vi "Auto2.vi"() -> ()   [LabVIEW 2020]
uses:
  Global_Variable/A180648.vi
  Global_Variable/Global.vi
  Global_Variable/excursion.vi
  <userlib>/_MGI/1D Array/MGI Running Average/MGI Running Average(DBL).vi
  <userlib>/_MGI/1D Array/MGI Average/MGI Average (DBL[][]).vi
  Libraries/S7/S7.lvlib
  <vilib>/ptbypt/NI_PtbyPt.lvlib
panel:
  out "合格状态":bool
  out "可信度检测":cluster{dbl[], dbl[]}[](graph)
  out "传感器特性":cluster{dbl[], dbl[]}[](graph)
  out "初始角度":dbl
  out "T1-T2_135°":dbl
  out "T1-T2_225°":dbl
  out "T1-T2_315°":dbl
  out "T1-T2_360°":dbl
  out "T1-T2_270°":dbl
  out "T1-T2_180°":dbl
  out "T1-T2_45°":dbl
  out "T1-T2_90°":dbl
  out "初始化 3":bool[](array[boolean])
  out "动优化态前":cluster{dbl[], dbl[]}[](graph)
  in  "initialize 2":bool caption="初始化"
  in  "initialize":bool caption="初始化"
  out "vRES_cCW":cluster{dbl[], dbl[]}
  out "VRES_cW":cluster{dbl[], dbl[]}
  out "初始化 2":bool[](array[boolean])
  in  "选项卡控件":enum32{"工位二程序复检", "工位二动态复检"}(tab)
  in  "请启动":bool
  out "Vres_45°":dbl format="%#.6f"
  out "Vres_135°":dbl format="%#.6f"
  out "Vres_225°":dbl format="%#.6f"
  out "Vres_315°":dbl format="%#.6f"
  out "Vres_360°":dbl format="%#.6f"
  out "Vres_270°":dbl format="%#.6f"
  out "Vres_180°":dbl format="%#.6f"
  out "Vres_90°":dbl format="%#.6f"
  out "S_CCw":dbl[](array[numeric]) caption="数据" format="%0.6f"
  out "P_CCw":dbl[](array[numeric]) caption="数据" format="%0.6f"
  out "S_CW":dbl[](array[numeric]) caption="数据" format="%0.6f"
  out "P_CW":dbl[](array[numeric]) caption="数据" format="%0.6f"
  out "T1_CCw":dbl[](array[numeric]) caption="数据" format="%0.2f"
  out "T2_CCw":dbl[](array[numeric]) caption="数据" format="%0.2f"
  out "T2_CW":dbl[](array[numeric]) caption="数据" format="%0.2f"
  out "T1_CW":dbl[](array[numeric]) caption="数据" format="%0.2f"
  out "初始化":bool[](array[boolean])
  out "SENSOR":T1
  in  "判定结果":bool[][](array[boolean])=[[TRUE]]
  in  "STEP":string
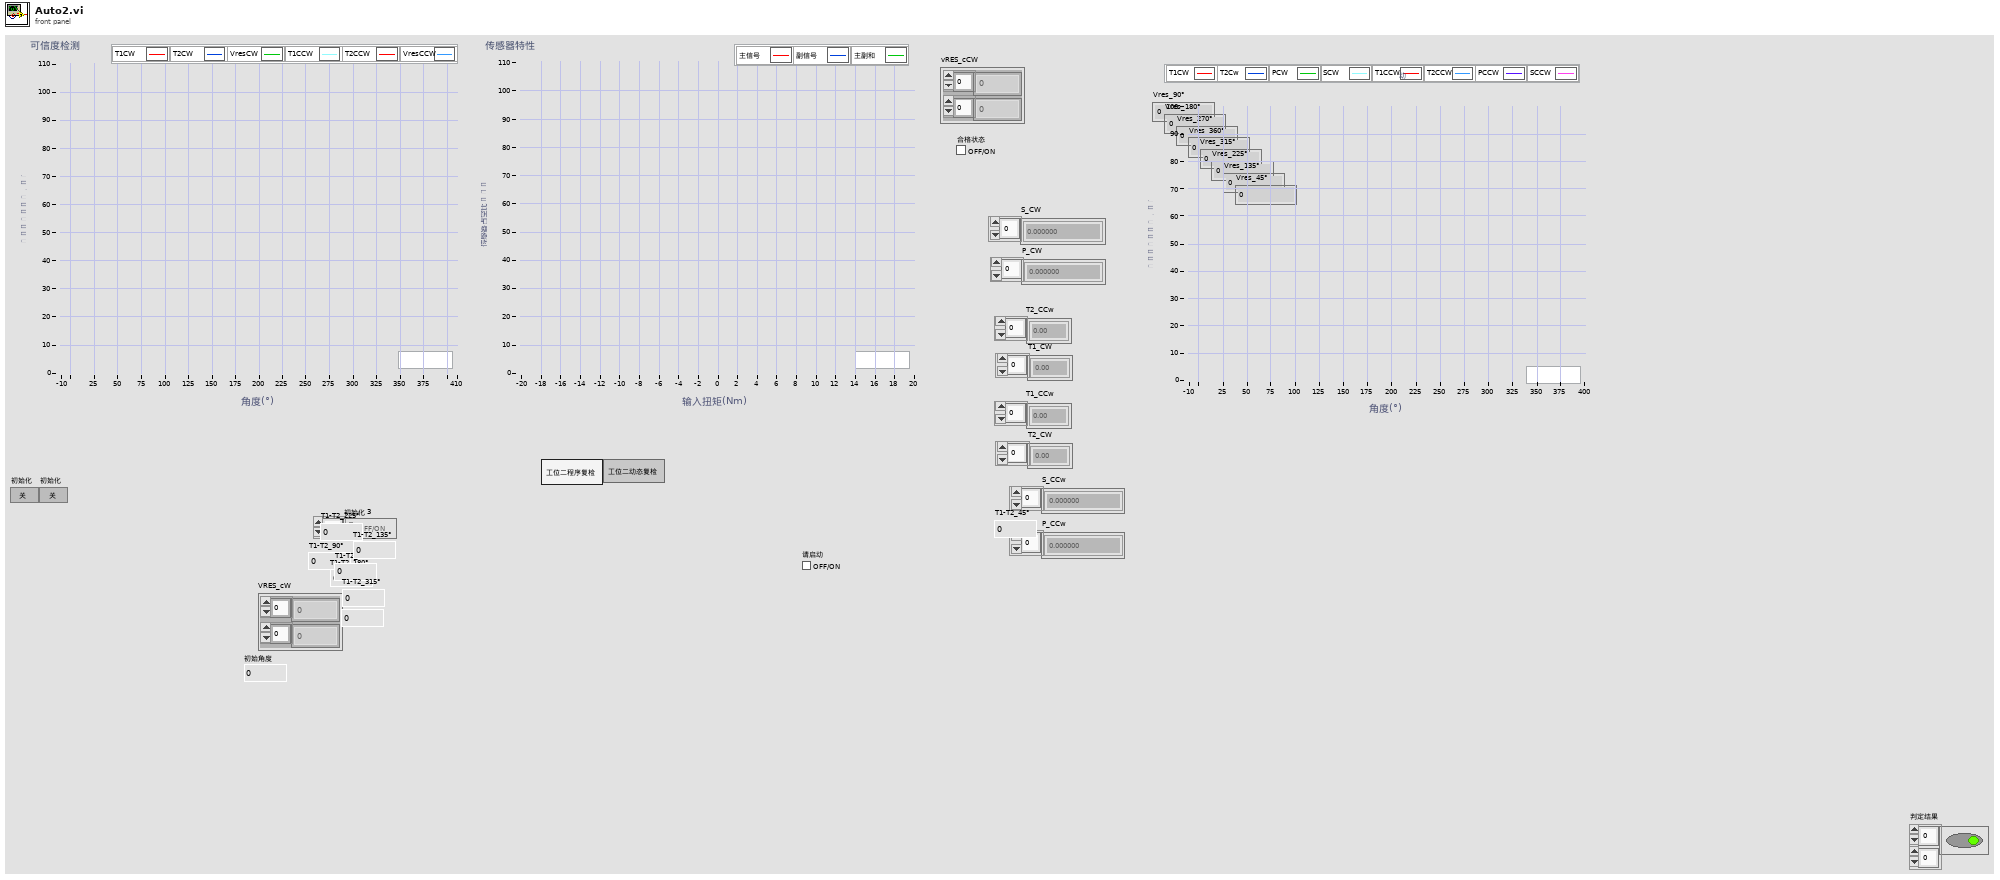
[diagram p1: front panel]
types:
  T1 = cluster{"hSENSOR":i32, "hASIC_T1":i32, "hASIC_T2":i32, "hASIC_P":i32, "hASIC_S":i32}
  T2 = typedef "检测CTR.xctl/检测CTR数据.ctl" = enum16{"Idle", "Runing", "Pass", "Faild", "Skip"}
  T3 = enum32{"Invalid", "Standard", "Closed", "Hidden", "Minimized", "Maximized"}
  T4 = enum16{"Idle", "Runing", "Pass", "Faild", "Skip"}
  T5 = enum16{"open", "replace", "create", "open or create", "replace or create", "replace or create with confirmation"}
  T6 = cluster{"工位一驱动伺服位移":sgl, "工位二驱动伺服位移":sgl, "工位一移载伺服位移":sgl, "工位二移载伺服位移":sgl, "工位一编码器位移":sgl, "工位二编码器位移":sgl, "工位一扭矩":sgl, "工位二扭矩":sgl}
  T7 = typedef "System_conf.ctl" = cluster{"右上升":dbl, "右下降":dbl, "左上升":dbl, "左下降":dbl, "左逆向":dbl, "左正向":dbl}
  T8 = cluster{"主副信号和MAX":cluster{"单位":string, "下限":dbl, "上限":dbl}, "主副信号和MIN":cluster{"单位":string, "下限":dbl, "上限":dbl}, "主信号线性误差":cluster{"单位":string, "下限":dbl, "上限":dbl}, "副信号线性误差":cluster{"单位":string, "下限":dbl, "上限":dbl}, "主信号MAX":cluster{"单位":string, "下限":dbl, "上限":dbl}, "主信号MIN":cluster{"单位":string, "下限":dbl, "上限":dbl}, "副信号MAX":cluster{"单位":string, "下限":dbl, "上限":dbl}, "副信号MIN":cluster{"单位":string, "下限":dbl, "上限":dbl}, "中心偏移量":cluster{"单位":string, "下限":dbl, "上限":dbl}, "定点设置":cluster{"单位":string, "下限":dbl, "上限":dbl}, "定点左侧主信号":cluster{"单位":string, "下限":dbl, "上限":dbl}, "定点左侧副信号":cluster{"单位":string, "下限":dbl, "上限":dbl}, "定点右侧主信号":cluster{"单位":string, "下限":dbl, "上限":dbl}, "定点右侧副信号":cluster{"单位":string, "下限":dbl, "上限":dbl}, "监测点1左滞后":cluster{"单位":string, "下限":dbl, "上限":dbl}, "监测点1右滞后":cluster{"单位":string, "下限":dbl, "上限":dbl}, "监测点2左滞后":cluster{"单位":string, "下限":dbl, "上限":dbl}, "监测点2右滞后":cluster{"单位":string, "下限":dbl, "上限":dbl}, "监测点3左滞后":cluster{"单位":string, "下限":dbl, "上限":dbl}, "监测点3右滞后":cluster{"单位":string, "下限":dbl, "上限":dbl}}
  T9 = cluster{"复检速度":dbl, "换向扭矩":dbl, "判定范围下限":dbl, "判定范围上限":dbl, "滞后监测点1":dbl, "滞后监测点2":dbl, "滞后监测点3":dbl}
  T10 = cluster{"可信度检测":cluster{dbl[], dbl[]}[], "动优化态前":cluster{dbl[], dbl[]}[], "传感器特性":cluster{dbl[], dbl[]}[]}
  T11 = typedef "lveventtype.ctl" = enum32{"Null", "Timeout", "Annotation Menu Selection", "Annotation Menu Selection?", "App Instance Close", "App Instance Close?", "Autoscale Range Change", "Bookmark Info Change", "Cell Edit", "Cell Edit?", "Cursor Grab", "Cursor Grab?", "Cursor Menu Selection", "Cursor Menu Selection?", "Cursor Move", "Cursor Release", "Data Change", "Direction Change", "Display State Change", "Drag Ended", "Drag Enter", "Drag Leave", "Drag Over", "Drag Source Update", "Drag Starting", "Drag Starting?", "Drop", "Exec State Change", "Key Down", "Key Down?", "Key Repeat", "Key Repeat?", "Key Up", "Listbox Double Click", "Menu Activation?", "Menu Selection (App)", "Menu Selection? (App)", "Menu Selection (User)", "Mouse Down", "Mouse Down?", "Mouse Enter", "Mouse Leave", "Mouse Move", "Mouse Up", "Mouse Wheel", "NI Security User Change (App)", "Pane Size", "Panel Close", "Panel Close?", "Panel Resize", "Plot Attribute Change", "Scale Range Change", "Shortcut Menu Activation?", "Shortcut Menu Selection (App)", "Shortcut Menu Selection? (App)", "Shortcut Menu Selection (User)", "Tree Double Click", "Tree Drag", "Tree Drag?", "Tree Drop", "Tree Drop?", "Tree Item Close", "Tree Item Close?", "Tree Item Open", "Tree Item Open?", "User Event", "Value Change"}
  T12 = typedef "LVPoint32TypeDef.ctl" = cluster{"Horizontal":i32, "Vertical":i32}
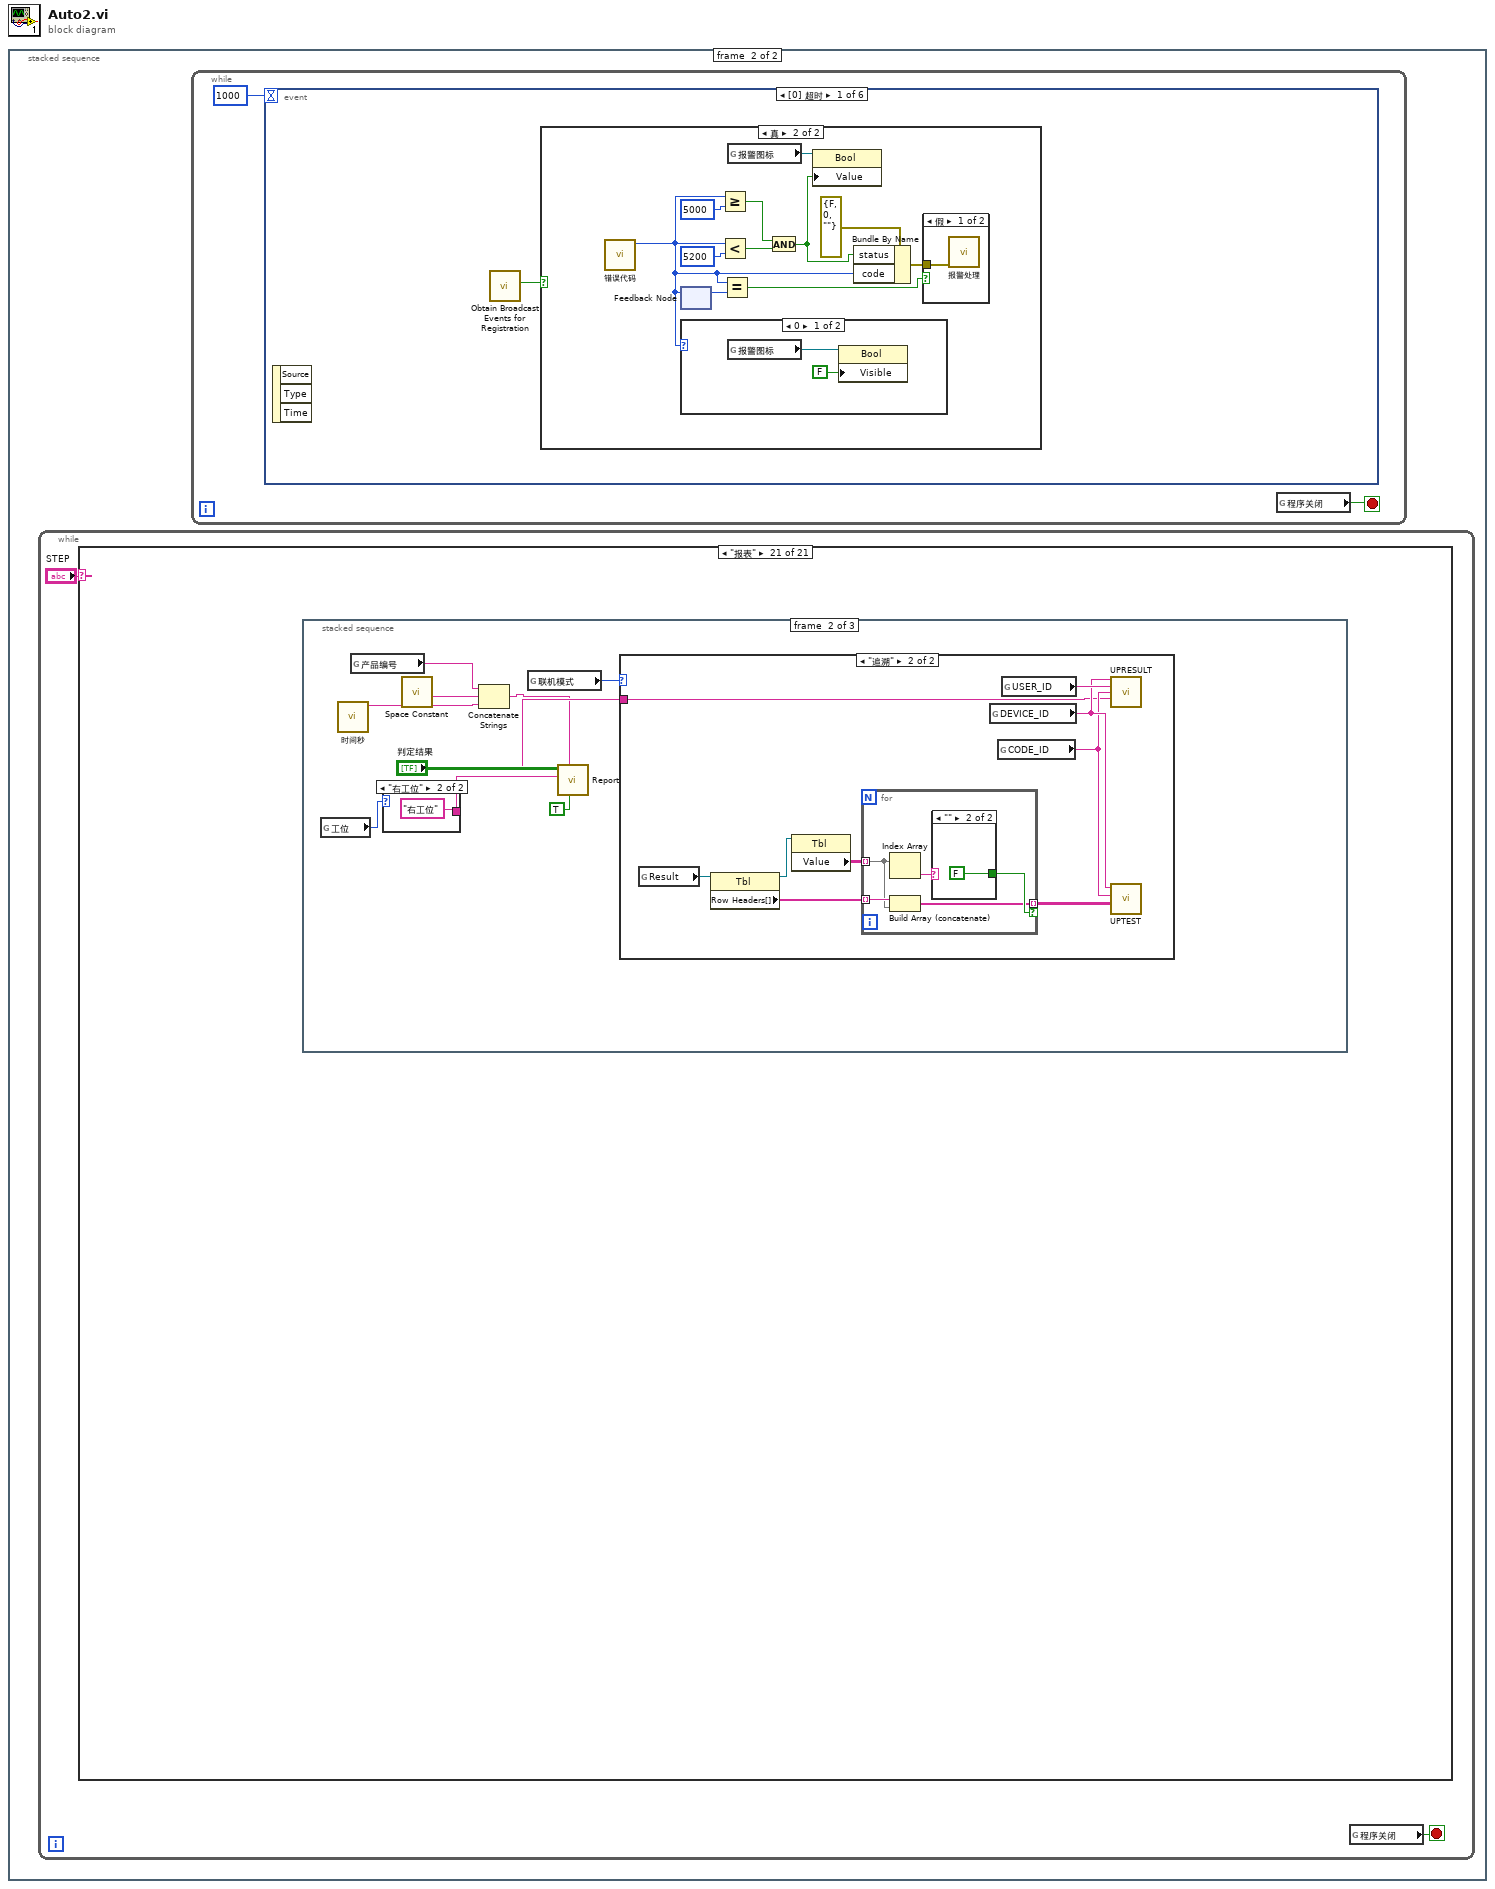
[diagram p0: block diagram]
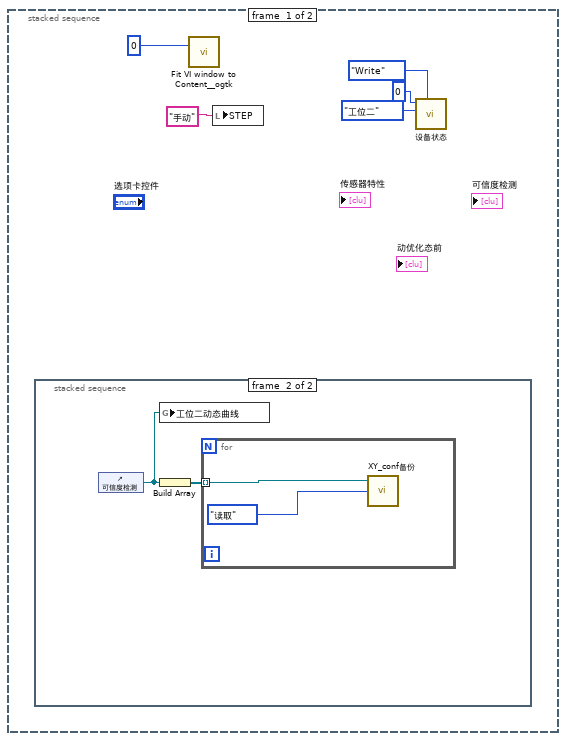
[diagram p2: hidden frame]
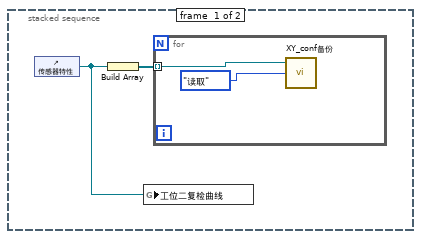
[diagram p3: hidden frame]
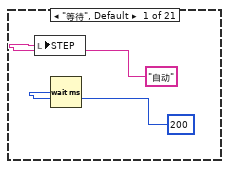
[diagram p4: hidden frame]
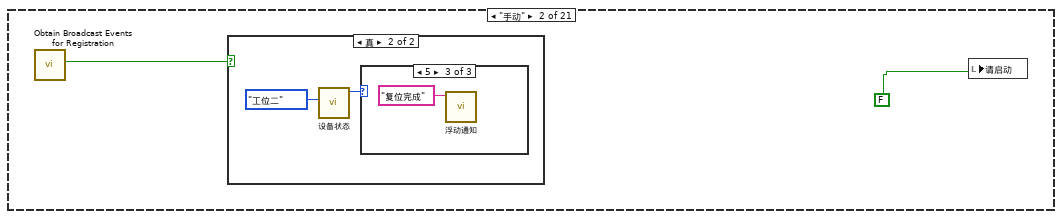
[diagram p5: hidden frame]
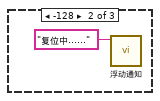
[diagram p8: hidden frame]
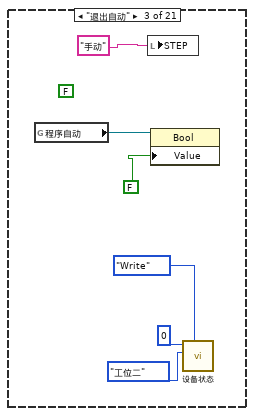
[diagram p9: hidden frame]
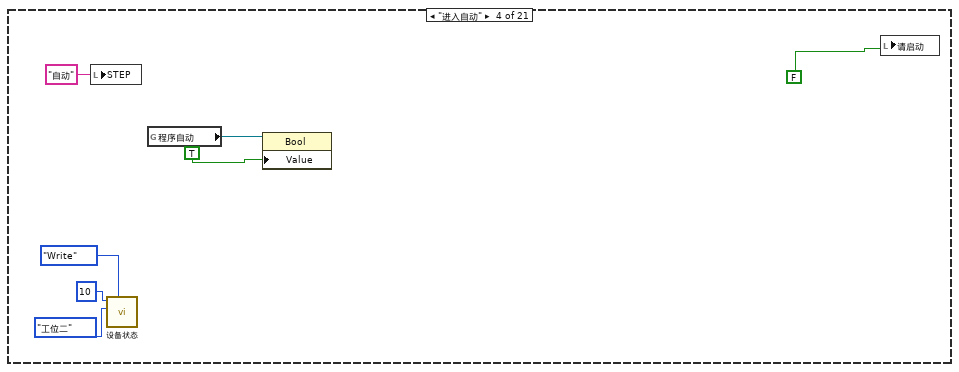
[diagram p10: hidden frame]
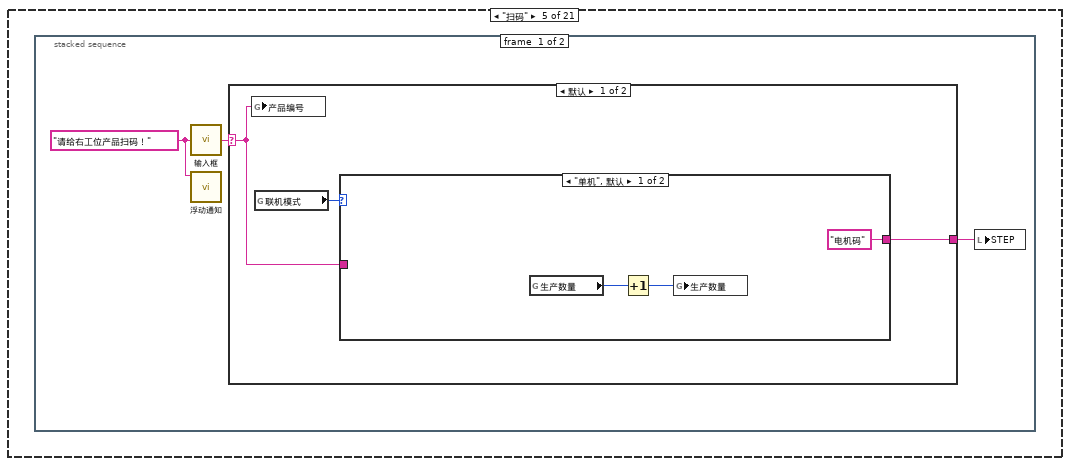
[diagram p11: hidden frame]
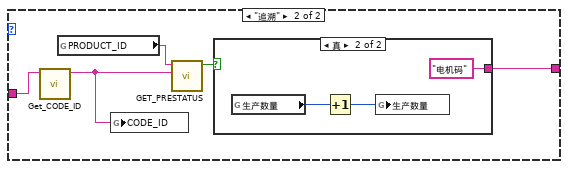
[diagram p12: hidden frame]
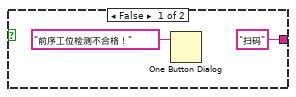
[diagram p13: hidden frame]
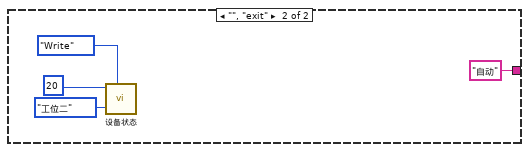
[diagram p14: hidden frame]
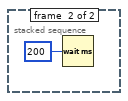
[diagram p15: hidden frame]
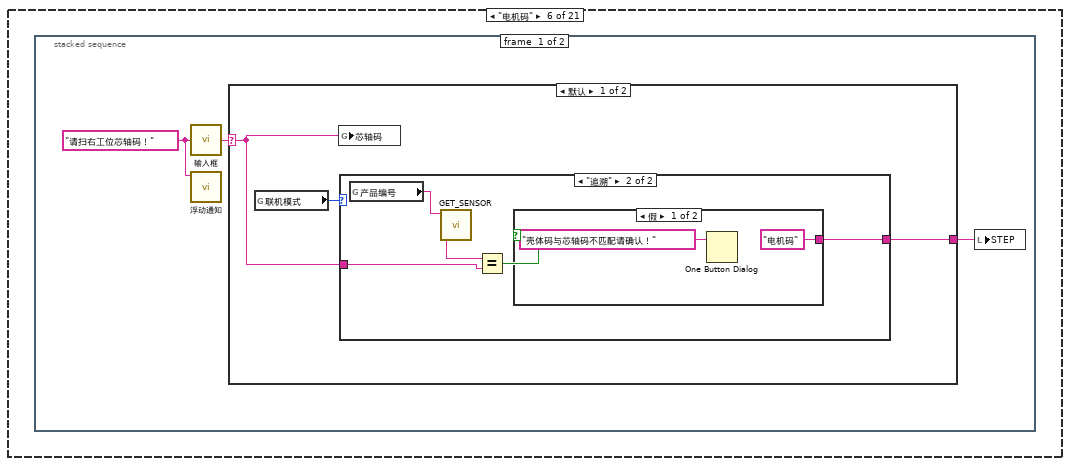
[diagram p16: hidden frame]
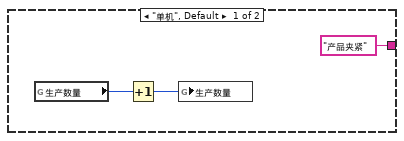
[diagram p17: hidden frame]
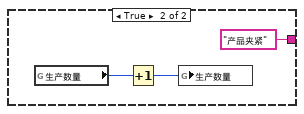
[diagram p18: hidden frame]
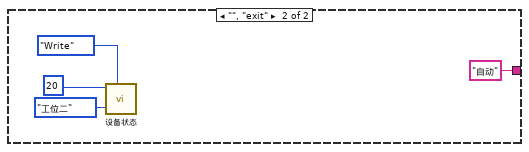
[diagram p19: hidden frame]
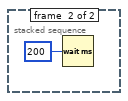
[diagram p20: hidden frame]
diagram:
  n1 = stacked-sequence {
    frame #0 {
      n2 = stacked-sequence {
        frame #0 {
          n3 = control-ref of="传感器特性"() -> (w6:refnum<vi>)
          n4 = Build Array(w6) -> (w7:refnum<vi>[])
          n5 = global write "A180648.vi" "工位二复检曲线"(w6) -> ()
          n6 = for "For循环" {
            tunnel: w7 -> [w8] mode=indexing
            n7 = call "XY_conf备份.vi"("方式"=enum16{"写入", "读取"}."读取", "XY图引用"=w8) -> ()  [unwired: 3 in, 1 out]
          }
        }
        frame #1 {
          n8 = control-ref of="可信度检测"() -> (w11:refnum<vi>)
          n9 = global write "A180648.vi" "工位二动态曲线"(w11) -> ()
          n10 = Build Array(w11) -> (w10:refnum<vi>[])
          n11 = for "For循环" {
            tunnel: w10 -> [w12] mode=indexing
            n12 = call "XY_conf备份.vi"("方式"=enum16{"写入", "读取"}."读取", "XY图引用"=w12) -> ()  [unwired: 3 in, 1 out]
          }
        }
      }
      n13 = call <userlib>:"Fit VI window to Content__ogtk.vi"("border spacing (2 px)"=0) -> ()  [unwired: 5 in, 2 out]
      n14 = local write "STEP"("手动" ("STEP")) -> ()
      n15 = call "设备状态.vi"("枚举"=enum16{"Read", "Write"}."Write", "工位"=enum16{"工位一", "工位二"}."工位二", "Status_Write"=i16 0) -> ()  [unwired: 8 in, 1 out]
    }
    frame #1 {
      n16 = while {
        stop <- w15 stop-if-true
        n17 = case shown="\"报表\"" "STEP" {
          frame "等待", Default {
            n18 = local write "STEP"("自动" ("STEP")) -> ()
            n19 = Wait (ms)(milliseconds to wait=u32 200 ("等待时间（毫秒）")) -> ()  [unwired: 1 out]
          }
          frame "手动" {
            n20 = call "Obtain Broadcast Events for Registration.vi"() -> ("Already running?"=w19:bool)  [unwired: 9 in, 2 out]
            n21 = case shown="真" w19 {
              frame False {
              }
              frame True {
                n22 = call "设备状态.vi"("工位"=enum16{"工位一", "工位二"}."工位二") -> ("Status_Read"=w21:i16)  [unwired: 10 in]
                n23 = case shown="5" w21 {
                  frame 0, Default {
                  }
                  frame -128 {
                    n24 = call "浮动通知.vi"("通知内容"="复位中……" ("Status")) -> ()  [unwired: 11 in]
                  }
                  frame 5 {
                    n25 = call "浮动通知.vi"("通知内容"="复位完成" ("Status")) -> ()  [unwired: 11 in]
                  }
                }
              }
            }
            n26 = local write "请启动"(FALSE ("请启动")) -> ()
          }
          frame "退出自动" {
            (unwired) FALSE ("计时开始")
            n27 = global read "Global.vi" "程序自动"() -> (w26:refnum<vi>)
            n28 = local write "STEP"("手动" ("STEP")) -> ()
            n29 = property class="Bool"(reference=w26, "Value"=FALSE) -> ()  [unwired: 1 in, 2 out]
            n30 = call "设备状态.vi"("枚举"=enum16{"Read", "Write"}."Write", "工位"=enum16{"工位一", "工位二"}."工位二", "Status_Write"=i16 0) -> ()  [unwired: 8 in, 1 out]
          }
          frame "进入自动" {
            n31 = local write "STEP"("自动" ("STEP")) -> ()
            n32 = call "设备状态.vi"("枚举"=enum16{"Read", "Write"}."Write", "工位"=enum16{"工位一", "工位二"}."工位二", "Status_Write"=i16 10) -> ()  [unwired: 8 in, 1 out]
            n33 = global read "Global.vi" "程序自动"() -> (w35:refnum<vi>)
            n34 = property class="Bool"(reference=w35, "Value"=TRUE) -> ()  [unwired: 1 in, 2 out]
            n35 = local write "请启动"(FALSE ("请启动")) -> ()
          }
          frame "扫码" {
            n36 = stacked-sequence {
              frame #0 {
                w38 = "请给右工位产品扫码！" ("提示信息")
                n37 = call "输入框.vi"("提示信息"=w38) -> ("条形码输出"=w39:string)
                n38 = call "浮动通知.vi"("通知内容"=w38) -> ()  [unwired: 11 in]
                n39 = case shown="默认" w39 {
                  selector: w39 -> [w40 _]
                  tunnel: [w42 "自动" ("State(s) in Front (\"\")")] -> w37
                  frame Default {
                    n40 = global write "Global.vi" "产品编号"(w40) -> ()
                    n41 = global read "Global.vi" "联机模式"() -> (w41:enum16{"单机", "追溯"})
                    n42 = case shown="\"单机\", 默认" w41 {
                      tunnel: ["电机码" ("State(s) in Front (\"\")") w50] -> w42
                      tunnel: w40 -> [_ w47]
                      frame "单机", Default {
                        n43 = global read "Global.vi" "生产数量"() -> (w43:i32)
                        n44 = Increment(x=w43) -> (x+1=w44:i32)
                        n45 = global write "Global.vi" "生产数量"(w44) -> ()
                      }
                      frame "追溯" {
                        n46 = call "Get_CODE_ID.vi"("CODE_MAIN"=w47) -> ("CODE_ID"=w46:string)  [unwired: 10 in]
                        n47 = global read "追溯Global.vi" "PRODUCT_ID"() -> (w49:string)
                        n48 = global write "追溯Global.vi" "CODE_ID"(w46) -> ()
                        n49 = call "GET_PRESTATUS.vi"("CODE_ID"=w46, "PRODUCT_ID"=w49) -> ("OK?"=w48:bool)  [unwired: 9 in]
                        n50 = case shown="真" w48 {
                          tunnel: ["扫码" ("State(s) in Front (\"\")") "电机码" ("State(s) in Front (\"\")")] -> w50
                          frame False {
                            n51 = One Button Dialog(message="前序工位检测不合格！" ("消息")) -> ()  [unwired: 1 in, 1 out]
                          }
                          frame True {
                            n52 = global read "Global.vi" "生产数量"() -> (w53:i32)
                            n53 = Increment(x=w53) -> (x+1=w54:i32)
                            n54 = global write "Global.vi" "生产数量"(w54) -> ()
                          }
                        }
                      }
                    }
                  }
                  frame "", "exit" {
                    n55 = call "设备状态.vi"("枚举"=enum16{"Read", "Write"}."Write", "工位"=enum16{"工位一", "工位二"}."工位二", "Status_Write"=i16 20) -> ()  [unwired: 8 in, 1 out]
                  }
                }
                n56 = local write "STEP"(w37) -> ()
              }
              frame #1 {
                n57 = Wait (ms)(milliseconds to wait=u32 200 ("等待时间（毫秒）")) -> ()  [unwired: 1 out]
              }
            }
          }
          frame "电机码" {
            n58 = stacked-sequence {
              frame #0 {
                w62 = "请扫右工位芯轴码！" ("提示信息")
                n59 = call "输入框.vi"("提示信息"=w62) -> ("条形码输出"=w63:string)
                n60 = call "浮动通知.vi"("通知内容"=w62) -> ()  [unwired: 11 in]
                n61 = case shown="默认" w63 {
                  selector: w63 -> [w64 _]
                  tunnel: [w66 "自动" ("State(s) in Front (\"\")")] -> w61
                  frame Default {
                    n62 = global read "Global.vi" "联机模式"() -> (w65:enum16{"单机", "追溯"})
                    n63 = global write "Global.vi" "芯轴码"(w64) -> ()
                    n64 = case shown="\"追溯\"" w65 {
                      tunnel: ["产品夹紧" ("State(s) in Front (\"\")") w74] -> w66
                      tunnel: w64 -> [_ w72]
                      frame "单机", Default {
                        n65 = global read "Global.vi" "生产数量"() -> (w67:i32)
                        n66 = Increment(x=w67) -> (x+1=w68:i32)
                        n67 = global write "Global.vi" "生产数量"(w68) -> ()
                      }
                      frame "追溯" {
                        n68 = global read "Global.vi" "产品编号"() -> (w70:string)
                        n69 = call "GET_SENSOR.vi"("CODE_MAIN"=w70) -> ("CODE_MOTOR"=w73:string)  [unwired: 10 in]
                        n70 = Equal?(x=w73, y=w72) -> (x = y?=w71:bool)
                        n71 = case shown="假" w71 {
                          tunnel: ["电机码" ("State(s) in Front (\"\")") "产品夹紧" ("State(s) in Front (\"\")")] -> w74
                          frame False {
                            n72 = One Button Dialog(message="壳体码与芯轴码不匹配请确认！" ("消息")) -> ()  [unwired: 1 in, 1 out]
                          }
                          frame True {
                            n73 = global read "Global.vi" "生产数量"() -> (w77:i32)
                            n74 = Increment(x=w77) -> (x+1=w78:i32)
                            n75 = global write "Global.vi" "生产数量"(w78) -> ()
                          }
                        }
                      }
                    }
                  }
                  frame "", "exit" {
                    n76 = call "设备状态.vi"("枚举"=enum16{"Read", "Write"}."Write", "工位"=enum16{"工位一", "工位二"}."工位二", "Status_Write"=i16 20) -> ()  [unwired: 8 in, 1 out]
                  }
                }
                n77 = local write "STEP"(w61) -> ()
              }
              frame #1 {
                n78 = Wait (ms)(milliseconds to wait=u32 200 ("等待时间（毫秒）")) -> ()  [unwired: 1 out]
              }
            }
          }
          frame "传感器码" {
            n79 = stacked-sequence {
              frame #0 {
                w86 = "请给右工位产品扫码！" ("提示信息")
                n80 = call "输入框.vi"("提示信息"=w86) -> ("条形码输出"=w87:string)
                n81 = call "浮动通知.vi"("通知内容"=w86) -> ()  [unwired: 11 in]
                n82 = case shown="默认" w87 {
                  selector: w87 -> [w88 _]
                  tunnel: [w90 "自动" ("State(s) in Front (\"\")")] -> w85
                  frame Default {
                    n83 = global write "Global.vi" "产品编号"(w88) -> ()
                    n84 = global read "Global.vi" "联机模式"() -> (w89:enum16{"单机", "追溯"})
                    n85 = case shown="\"追溯\"" w89 {
                      tunnel: ["产品夹紧" ("State(s) in Front (\"\")") w98] -> w90
                      tunnel: w88 -> [_ w95]
                      frame "单机", Default {
                        n86 = global read "Global.vi" "生产数量"() -> (w91:i32)
                        n87 = Increment(x=w91) -> (x+1=w92:i32)
                        n88 = global write "Global.vi" "生产数量"(w92) -> ()
                      }
                      frame "追溯" {
                        n89 = call "Get_CODE_ID_Sensor.vi"("CODE_SENSOR"=w95) -> ("CODE_ID"=w94:string)  [unwired: 10 in]
                        n90 = global read "追溯Global.vi" "PRODUCT_ID"() -> (w97:string)
                        n91 = global write "追溯Global.vi" "CODE_ID"(w94) -> ()
                        n92 = call "GET_PRESTATUS.vi"("CODE_ID"=w94, "PRODUCT_ID"=w97) -> ("OK?"=w96:bool)  [unwired: 9 in]
                        n93 = case shown="假" w96 {
                          tunnel: ["传感器码" ("State(s) in Front (\"\")") "产品夹紧" ("State(s) in Front (\"\")")] -> w98
                          frame False {
                            n94 = One Button Dialog(message="前序工位检测不合格！" ("消息")) -> ()  [unwired: 1 in, 1 out]
                          }
                          frame True {
                            n95 = global read "Global.vi" "生产数量"() -> (w101:i32)
                            n96 = Increment(x=w101) -> (x+1=w102:i32)
                            n97 = global write "Global.vi" "生产数量"(w102) -> ()
                          }
                        }
                      }
                    }
                  }
                  frame "", "exit" {
                    n98 = call "设备状态.vi"("枚举"=enum16{"Read", "Write"}."Write", "工位"=enum16{"工位一", "工位二"}."工位二", "Status_Write"=i16 20) -> ()  [unwired: 8 in, 1 out]
                  }
                }
                n99 = local write "STEP"(w85) -> ()
              }
              frame #1 {
                n100 = Wait (ms)(milliseconds to wait=u32 200 ("等待时间（毫秒）")) -> ()  [unwired: 1 out]
              }
            }
          }
          frame "产品夹紧" {
            n101 = stacked-sequence {
              frame #0 {
                n102 = case shown="假" "请启动" {
                  frame False {
                    n103 = call "浮动通知.vi"("通知内容"="请启动右工位" ("Status")) -> ()  [unwired: 11 in]
                    n104 = call "设备状态.vi"("枚举"=enum16{"Read", "Write"}."Write", "工位"=enum16{"工位一", "工位二"}."工位二", "Status_Write"=i16 99) -> ()  [unwired: 8 in, 1 out]
                    n105 = local write "请启动"(TRUE ("请启动")) -> ()
                  }
                  frame True {
                  }
                }
              }
              frame #1 {
                n106 = call "设备状态.vi"("工位"=enum16{"工位一", "工位二"}."工位二") -> ("Status_Read"=w115:i16)  [unwired: 10 in]
                n107 = case shown="0, 默认" w115 {
                  frame 0, Default {
                  }
                  frame 100 {
                    n108 = local write "STEP"("初始化") -> ()
                    n109 = local write "请启动"(FALSE ("请启动")) -> ()
                  }
                }
              }
            }
          }
          frame "套输入轴" {
            n110 = global read "Global.vi" "可信度检测引用句柄"() -> (w125:refnum<vi>)
            n111 = global read "Global.vi" "传感器特性用句柄"() -> (w128:refnum<vi>)
            n112 = property class="检测CTR"(reference=w125) -> ("Value"=w126:variant)  [unwired: 1 in, 2 out]
            n113 = property class="检测CTR"(reference=w128) -> ("Value"=w127:variant)  [unwired: 1 in, 2 out]
            n114 = Variant To Data(type=检测CTR数据."Idle" ("Data"), Variant=w126) -> (data=w124:T2)  [unwired: 1 in, 1 out]
            n115 = Variant To Data(type=检测CTR数据."Idle" ("Data"), Variant=w127) -> (data=w129:T2)  [unwired: 1 in, 1 out]
            n116 = Equal?(x=w124, y=检测CTR数据."Skip" ("Data")) -> (x = y?=w130:bool)
            n117 = Equal?(x=w129, y=检测CTR数据."Skip" ("Data")) -> (x = y?=w131:bool)
            n118 = And(x=w130, y=w131) -> (x .and. y?=w119:bool)
            n119 = case shown="假" w119 {
              frame False {
                n120 = stacked-sequence {
                  frame #0 {
                    n121 = call "浮动通知.vi"("通知内容"="右工位产品套输入轴" ("Status")) -> ()  [unwired: 11 in]
                    n122 = call "设备状态.vi"("枚举"=enum16{"Read", "Write"}."Write", "工位"=enum16{"工位一", "工位二"}."工位二", "Status_Write"=i16 112) -> ()  [unwired: 8 in, 1 out]
                    n123 = vi-ref "T1T2占空比.vi"() -> (w135:refnum<vi>)
                    n124 = call "CallVI.vi"("VI引用"=w135, "状态"=T3."Hidden") -> ()  [unwired: 12 in, 2 out]
                    n125 = vi-ref "PS采集.vi"() -> (w132:refnum<vi>)
                    n126 = call "CallVI.vi"("VI引用"=w132, "状态"=T3."Hidden") -> ()  [unwired: 12 in, 2 out]
                  }
                  frame #1 {
                    n127 = while {
                      stop <- w140 stop-if-true
                      n128 = call "设备状态.vi"("工位"=enum16{"工位一", "工位二"}."工位二") -> ("Status_Read"=w141:i16)  [unwired: 10 in]
                      n129 = case shown="0, 默认" w141 {
                        tunnel: [w143 TRUE] -> w140
                        frame 0, Default {
                          n130 = call "套输入轴时间"() -> ("Time has Elapsed"=w144:bool)  [unwired: 12 in, 7 out]
                          n131 = case shown="真" w144 {
                            tunnel: [FALSE TRUE] -> w143
                            frame False {
                            }
                            frame True {
                              n132 = call "浮动通知.vi"("通知内容"="工位二产品套输入轴超时" ("Status")) -> ()  [unwired: 11 in]
                            }
                          }
                        }
                        frame 113 {
                          n133 = local write "STEP"("动态优化") -> ()
                        }
                      }
                    }
                  }
                }
              }
              frame True {
                n134 = local write "STEP"("程序固化" ("STEP")) -> ()
              }
            }
          }
          frame "套输出轴" {
            n135 = global read "Global.vi" "传感器特性用句柄"() -> (w155:refnum<vi>)
            n136 = property class="检测CTR"(reference=w155) -> ("Value"=w154:variant)  [unwired: 1 in, 2 out]
            n137 = Variant To Data(type=检测CTR数据."Idle" ("Data"), Variant=w154) -> (data=w156:T2)  [unwired: 1 in, 1 out]
            n138 = Equal?(x=w156, y=检测CTR数据."Skip" ("Data")) -> (x = y?=w151:bool)
            n139 = case shown="假" w151 {
              frame False {
                n140 = stacked-sequence {
                  frame #0 {
                    n141 = call "设备状态.vi"("枚举"=enum16{"Read", "Write"}."Write", "工位"=enum16{"工位一", "工位二"}."工位二", "Status_Write"=i16 108) -> ()  [unwired: 8 in, 1 out]
                    n142 = call "浮动通知.vi"("通知内容"="右工位产品套输出轴" ("Status")) -> ()  [unwired: 11 in]
                  }
                  frame #1 {
                    n143 = while {
                      stop <- w161 stop-if-true
                      n144 = call "设备状态.vi"("工位"=enum16{"工位一", "工位二"}."工位二") -> ("Status_Read"=w162:i16)  [unwired: 10 in]
                      n145 = case shown="0, 默认" w162 {
                        tunnel: [w164 TRUE] -> w161
                        frame 0, Default {
                          n146 = call "套输出轴时间"() -> ("Time has Elapsed"=w165:bool)  [unwired: 12 in, 7 out]
                          n147 = case shown="真" w165 {
                            tunnel: [FALSE TRUE] -> w164
                            frame False {
                            }
                            frame True {
                              n148 = call "浮动通知.vi"("通知内容"="右工位产品套输出轴超时" ("Status")) -> ()  [unwired: 11 in]
                            }
                          }
                        }
                        frame 109 {
                          n149 = call "传感器数据.vi"() -> ("传感器读数"=w170:T6)  [unwired: 11 in]
                          n150 = local write "STEP"("程序复检") -> ()
                          n151 = Unbundle By Name(w170) -> ("工位二驱动伺服位移"=→"初始角度":sgl)
                        }
                      }
                    }
                  }
                }
              }
              frame True {
                n152 = local read "判定结果"() -> (w174:bool[][])
                n153 = Build Array (concatenate)(w174, bool[][] [[FALSE, TRUE]] ("判定结果")) -> (w175:bool[][])
                n154 = local write "判定结果"(w175) -> ()
                n155 = local write "STEP"("程序固化" ("STEP")) -> ()
              }
            }
          }
          frame "初始化" {
            n156 = stacked-sequence {
              frame #0 {
                w182 = cluster{dbl[], dbl[]} {[], []} ("vRES_cCW")
                w180 = TRUE ("IO_Stop")
                n157 = global read "Global.vi" "产品型号"() -> (w178:string)
                n158 = global write "Global.vi" "IO_Stop"(w180) -> ()
                n159 = global write "Global.vi" "计时开始"(w180) -> ()
                n160 = global write "Global.vi" "工位占空比采集"(FALSE ("工位二占空比采集")) -> ()
                n161 = global write "Global.vi" "P/S采集"(FALSE ("工位二占空比采集")) -> ()
                n162 = local write "判定结果"(bool[][] [] ("判定结果")) -> ()
                n163 = call "System_Conf_RW.vi"("Mode"=enum16{"Read", "Write"}."Read", "Section"=w178) -> ("excursion_out"=w177:T7)  [unwired: 8 in, 1 out]
                n164 = global write "excursion.vi" "excursion"(w177) -> ()
                n165 = global write "Global.vi" "动态优化完成"(FALSE ("动态优化完成")) -> ()
                n166 = local write "vRES_cCW"(w182) -> ()
                n167 = local write "VRES_cW"(w182) -> ()
              }
              frame #1 {
                w191 = dbl[] [] ("S_CCw")
                w192 = dbl[] [] ("T1_cw")
                n168 = local write "T1_CW"(w192) -> ()
                n169 = local write "T2_CW"(w192) -> ()
                n170 = local write "P_CW"(w192) -> ()
                n171 = local write "P_CCw"(w192) -> ()
                n172 = for "For循环" {
                  N: 12 -> [_]
                  tunnel: [cluster{dbl[], dbl[]} {[], []}] -> w190 mode=indexing
                }
                n173 = local write "传感器特性"(w190) -> ()
                n174 = local write "S_CCw"(w191) -> ()
                n175 = local write "S_CW"(w191) -> ()
                n176 = local write "T1_CCw"(w191) -> ()
                n177 = local write "T2_CCw"(w191) -> ()
                n178 = for "For循环" {
                  N: 8 -> [_]
                  tunnel: [cluster{dbl[], dbl[]} {[], []}] -> w188 mode=indexing
                }
                n179 = for "For循环" {
                  N: 8 -> [_]
                  tunnel: [cluster{dbl[], dbl[]} {[], []}] -> w187 mode=indexing
                }
                n180 = local write "动优化态前"(w187) -> ()
                n181 = local write "可信度检测"(w188) -> ()
              }
              frame #2 {
                n182 = global read "Global.vi" "Result"() -> (w208:refnum<vi>)
                n183 = property class="Tbl"(reference=w208, "Value"=string[][] []) -> (reference out=w209:refnum<vi>, error out=w210:errorcluster)  [unwired: 1 in]
                n184 = property class="Tbl"(reference=w209, error in=w210, "Row Headers[]"=string[] [] ("列首字符串[]")) -> ()  [unwired: 2 out]
                n185 = Initialize Array(TRUE, 12 ("维数大小")) -> (→"初始化":bool[])
                n186 = Initialize Array(TRUE, 8 ("维数大小")) -> (→"初始化 2":bool[])
                n187 = Initialize Array(TRUE, 8 ("维数大小")) -> (→"初始化 3":bool[])
              }
              frame #3 {
                n188 = global read "Global.vi" "传感器特性用句柄"() -> (w214:refnum<vi>)
                n189 = global read "Global.vi" "可信度检测引用句柄"() -> (w211:refnum<vi>)
                n190 = global read "Global.vi" "动态优化引用句柄"() -> (w212:refnum<vi>)
                n191 = global read "Global.vi" "静态标定引用句柄"() -> (w216:refnum<vi>)
                n192 = global read "Global.vi" "程序固化引用句柄"() -> (w215:refnum<vi>)
                n193 = Build Array(w216, w215, w214, w212, w211) -> (w213:refnum<vi>[])
                n194 = for "For循环" {
                  tunnel: w213 -> [w226] mode=indexing
                  n195 = property class="检测CTR"(reference=w226) -> (reference out=w225:refnum<vi>, "Value"=w224:variant)  [unwired: 1 in, 1 out]
                  n196 = Variant To Data(type=检测CTR数据."Idle" ("Data"), Variant=w224) -> (data=w222:T2)  [unwired: 1 in, 1 out]
                  n197 = Equal?(x=w222, y=检测CTR数据."Skip" ("Data")) -> (x = y?=w220:bool)
                  n198 = Select(t=检测CTR数据."Skip" ("Data"), s=w220, f=检测CTR数据."Idle" ("Data")) -> (s? t:f=w217:T2)
                  n199 = property class="检测CTR"(reference=w225, "Value"=w217) -> ()  [unwired: 1 in, 2 out]
                }
              }
              frame #4 {
                n200 = local write "STEP"("静态标定" ("STEP")) -> ()
              }
            }
          }
          frame "静态标定" {
            n201 = global read "Global.vi" "静态标定引用句柄"() -> (w232:refnum<vi>)
            n202 = property class="检测CTR"(reference=w232) -> ("Value"=w231:variant)  [unwired: 1 in, 2 out]
            n203 = Variant To Data(type=检测CTR数据."Idle" ("Data"), Variant=w231) -> (data=w233:T2)  [unwired: 1 in, 1 out]
            n204 = Equal?(x=w233, y=检测CTR数据."Skip" ("Data")) -> (x = y?=w228:bool)
            n205 = case shown="真" w228 {
              frame False {
                n206 = stacked-sequence {
                  tunnel: [_ _ w250] -> w234
                  frame #0 {
                    n207 = global read "Global.vi" "静态标定引用句柄"() -> (w236:refnum<vi>)
                    n208 = call "浮动通知.vi"("通知内容"="静态标定" ("Status")) -> ()  [unwired: 11 in]
                    n209 = property class="检测CTR"(reference=w236, "Value"=T4."Runing" ("值")) -> ()  [unwired: 1 in, 2 out]
                  }
                  frame #1 {
                    n210 = flat-sequence {
                      frame #0 {
                        n211 = call "采集切换.vi"("工位"=enum16{"工位一", "工位二"}."工位二", "采集方式"=enum16{"板卡采集", "PGI采集"}."PGI采集") -> ()  [unwired: 10 in]
                      }
                      frame #1 {
                        n212 = Wait (ms)(milliseconds to wait=u32 100 ("等待时间（毫秒）")) -> ()  [unwired: 1 out]
                      }
                    }
                  }
                  frame #2 {
                    n213 = call "InitPGI.vi"("DeviceNumber"=1) -> ("SENSOR"=w242:T1, "error out"=w243:errorcluster)  [unwired: 13 in]
                    "SENSOR" <- w242
                    n214 = call "InitProduct.vi"("SENSOR"=w242, "error in (no error)"=w243) -> ("error out"=w241:errorcluster)  [unwired: 12 in, 1 out]
                    n215 = call "StaticCalibration改.vi"("SENSOR"=w242, "error in (no error)"=w241) -> ("OK？"=w245:bool, "error out"=w247:errorcluster)  [unwired: 9 in, 3 out]
                    n216 = call "浮动通知.vi"("通知内容"="静态标定中..." ("Status")) -> ()  [unwired: 11 in]
                    n217 = call "Error Converter (ErrCode or Status).vi"("error in (no error)"=w247) -> ("error out"=w246:errorcluster)  [unwired: 10 in]
                    n218 = Unbundle By Name(w246) -> ("source"=w248:string)
                    n219 = case shown="假" w245 {
                      tunnel: [w258 "套输入轴"] -> w250
                      tunnel: w248 -> [w256 _]
                      frame False {
                        n220 = global read "Global.vi" "静态标定引用句柄"() -> (w265:refnum<vi>)
                        n221 = local read "判定结果"() -> (w252:bool[][])
                        n222 = Build Array (concatenate)(w252, bool[][] [[TRUE, FALSE]] ("判定结果")) -> (w253:bool[][])
                        n223 = property class="检测CTR"(reference=w265, "Value"=T4."Faild" ("值")) -> ()  [unwired: 1 in, 2 out]
                        n224 = local write "判定结果"(w253) -> ()
                        n225 = Concatenate Strings("静态标定失败,可能原因:" ("字符串"), w256, "建议旋转传感器后重新标定\n是否重新标定？" ("消息")) -> (w254:string)
                        n226 = Two Button Dialog(message=w254, 1:"否" ("F按钮名称（“取消”）"), 2:"是" ("T按钮名称（“确定”）")) -> (T button?=w261:bool)
                        n227 = Select(t="初始化" ("T按钮名称（“确定”）"), s=w261, f="报表" ("F按钮名称（“取消”）")) -> (s? t:f=w258:string)
                      }
                      frame True {
                        n228 = global read "Global.vi" "静态标定引用句柄"() -> (w270:refnum<vi>)
                        n229 = local read "判定结果"() -> (w266:bool[][])
                        n230 = Build Array (concatenate)(w266, bool[][] [[TRUE, TRUE]] ("判定结果")) -> (w268:bool[][])
                        n231 = local write "判定结果"(w268) -> ()
                        n232 = property class="检测CTR"(reference=w270, "Value"=T4."Pass" ("值")) -> ()  [unwired: 1 in, 2 out]
                      }
                    }
                  }
                }
                n233 = local write "STEP"(w234) -> ()
              }
              frame True {
                n234 = local write "STEP"("套输入轴") -> ()
                n235 = local read "判定结果"() -> (w272:bool[][])
                n236 = Build Array (concatenate)(w272, bool[][] [[FALSE, TRUE]] ("判定结果")) -> (w274:bool[][])
                n237 = local write "判定结果"(w274) -> ()
              }
            }
          }
          frame "动态优化" {
            n238 = global read "Global.vi" "可信度检测引用句柄"() -> (w280:refnum<vi>)
            n239 = property class="检测CTR"(reference=w280) -> ("Value"=w279:variant)  [unwired: 1 in, 2 out]
            n240 = Variant To Data(type=检测CTR数据."Idle" ("Data"), Variant=w279) -> (data=w281:T2)  [unwired: 1 in, 1 out]
            n241 = Equal?(x=w281, y=检测CTR数据."Skip" ("Data")) -> (x = y?=w276:bool)
            n242 = case shown="假" w276 {
              frame False {
                n243 = stacked-sequence {
                  frame #0 {
                    n244 = global read "Global.vi" "可信度检测引用句柄"() -> (w284:refnum<vi>)
                    n245 = call "浮动通知.vi"("通知内容"="可信度检测" ("Status")) -> ()  [unwired: 11 in]
                    n246 = property class="检测CTR"(reference=w284, "Value"=T4."Runing" ("值")) -> ()  [unwired: 1 in, 2 out]
                  }
                  frame #1 {
                    n247 = global read "Global.vi" "跳过优化"() -> (w286:bool)
                    n248 = case shown="真" w286 {
                      selector: w286 -> [_ w293]
                      tunnel: ["自动" w291] -> w285
                      frame False {
                        n249 = call "设备状态.vi"("枚举"=enum16{"Read", "Write"}."Write", "工位"=enum16{"工位一", "工位二"}."工位二", "Status_Write"=i16 505) -> ()  [unwired: 8 in, 1 out]
                      }
                      frame True {
                        n250 = global read "Global.vi" "动态优化复测"() -> (w292:bool)
                        n251 = global write "Global.vi" "动态优化完成"(w293) -> ()
                        n252 = case shown="真" w292 {
                          tunnel: [w294 "自动"] -> w291
                          frame False {
                            n253 = global read "Global.vi" "8点复测"() -> (w295:bool)
                            n254 = case shown="假" w295 {
                              tunnel: ["复测判定" "复测"] -> w294
                              frame False {
                              }
                              frame True {
                              }
                            }
                          }
                          frame True {
                            n255 = call "设备状态.vi"("枚举"=enum16{"Read", "Write"}."Write", "工位"=enum16{"工位一", "工位二"}."工位二", "Status_Write"=i16 505) -> ()  [unwired: 8 in, 1 out]
                          }
                        }
                      }
                    }
                    n256 = local write "STEP"(w285) -> ()
                  }
                }
              }
              frame True {
                n257 = local write "STEP"("套输出轴") -> ()
                n258 = local read "判定结果"() -> (w303:bool[][])
                n259 = Build Array (concatenate)(w303, bool[][] [[FALSE, TRUE]] ("判定结果")) -> (w304:bool[][])
                n260 = local write "判定结果"(w304) -> ()
              }
            }
          }
          frame "复测" {
            n261 = stacked-sequence {
              frame #0 {
                n262 = Wait (ms)(milliseconds to wait=u32 300 ("等待时间（毫秒）")) -> ()  [unwired: 1 out]
              }
              frame #1 {
                n263 = local write "STEP"("自动") -> ()
                n264 = call "浮动通知.vi"("通知内容"="复测" ("Status")) -> ()  [unwired: 11 in]
                n265 = call "设备状态.vi"("枚举"=enum16{"Read", "Write"}."Write", "工位"=enum16{"工位一", "工位二"}."工位二", "Status_Write"=i16 510) -> ()  [unwired: 8 in, 1 out]
              }
            }
          }
          frame "复测判定" {
            n266 = local read "Vres_90°"() -> (w332:dbl)
            n267 = local read "Vres_180°"() -> (w331:dbl)
            n268 = local read "Vres_270°"() -> (w330:dbl)
            n269 = local read "Vres_360°"() -> (w329:dbl)
            n270 = local read "Vres_315°"() -> (w324:dbl)
            n271 = local read "Vres_225°"() -> (w323:dbl)
            n272 = local read "Vres_135°"() -> (w322:dbl)
            n273 = local read "Vres_45°"() -> (w328:dbl)
            n274 = local read "T1-T2_90°"() -> (w321:dbl)
            n275 = local read "T1-T2_180°"() -> (w320:dbl)
            n276 = local read "T1-T2_270°"() -> (w319:dbl)
            n277 = local read "T1-T2_360°"() -> (w315:dbl)
            n278 = local read "T1-T2_315°"() -> (w316:dbl)
            n279 = local read "T1-T2_225°"() -> (w317:dbl)
            n280 = local read "T1-T2_135°"() -> (w318:dbl)
            n281 = local read "T1-T2_45°"() -> (w327:dbl)
            n282 = Build Array(w332, w331, w330, w329, w324, w323, w322, w328) -> (w313:dbl[])
            n283 = Build Array(w321, w320, w319, w315, w316, w317, w318, w327) -> (w326:dbl[])
            n284 = Absolute Value(x=w326) -> (abs(x)=w325:dbl[])
            n285 = call "CloseVI.vi"("名称或相对路径"="PS采集.vi") -> ()  [unwired: 10 in, 1 out]
            n286 = disable-structure shown="禁用" {
              frame Disabled {
                n287 = Two Button Dialog(message="复测失败\n请选择是否继续？" ("消息"), 1:"否" ("F按钮名称（“取消”）"), 2:"是" ("T按钮名称（“确定”）")) -> ()  [unwired: 1 out]
                n288 = case shown="真" {
                  selector: _ -> [_ _]
                  frame False {
                  }
                  frame True {
                    n289 = local write "STEP"("套输出轴" ("T按钮名称（“确定”）")) -> ()
                  }
                }
              }
              frame Enabled {
              }
            }
            n290 = call "动态优化复测判定2.vi"("T1-T2"=w325, "Vres"=w313) -> ("结果1"=w314:bool)  [unwired: 9 in]
            n291 = case shown="真" w314 {
              frame False {
                w339 = enum16{"Read", "Write"}."Write" ("枚举")
                w338 = enum16{"工位一", "工位二"}."工位二" ("工位")
                n292 = global read "Global.vi" "可信度检测引用句柄"() -> (w346:refnum<vi>)
                n293 = local read "判定结果"() -> (w342:bool[][])
                n294 = Build Array (concatenate)(w342, bool[][] [[TRUE, FALSE]] ("判定结果")) -> (w343:bool[][])
                n295 = local write "判定结果"(w343) -> ()
                n296 = property class="检测CTR"(reference=w346, "Value"=T4."Faild" ("值")) -> ()  [unwired: 1 in, 2 out]
                n297 = local write "STEP"("报表" ("F按钮名称（“取消”）")) -> ()
                n298 = call "设备状态.vi"("枚举"=w339, "工位"=w338, "Status_Write"=i16 400) -> ()  [unwired: 8 in, 1 out]
                n299 = call "合格状态.vi"("枚举"=w339, "工位"=w338, "Status_Write"=i16 2) -> ()  [unwired: 8 in, 1 out]
              }
              frame True {
                n300 = global read "Global.vi" "可信度检测引用句柄"() -> (w351:refnum<vi>)
                n301 = local read "判定结果"() -> (w347:bool[][])
                n302 = local write "STEP"("套输出轴") -> ()
                n303 = Build Array (concatenate)(w347, bool[][] [[TRUE, TRUE]] ("判定结果")) -> (w348:bool[][])
                n304 = local write "判定结果"(w348) -> ()
                n305 = property class="检测CTR"(reference=w351, "Value"=T4."Pass" ("值")) -> ()  [unwired: 1 in, 2 out]
              }
            }
          }
          frame "程序固化" {
            n306 = global read "Global.vi" "程序固化引用句柄"() -> (w357:refnum<vi>)
            n307 = property class="检测CTR"(reference=w357) -> ("Value"=w356:variant)  [unwired: 1 in, 2 out]
            n308 = Variant To Data(type=检测CTR数据."Idle" ("Data"), Variant=w356) -> (data=w358:T2)  [unwired: 1 in, 1 out]
            n309 = Equal?(x=w358, y=检测CTR数据."Skip" ("Data")) -> (x = y?=w353:bool)
            n310 = case shown="假" w353 {
              frame False {
                n311 = stacked-sequence {
                  frame #0 {
                    n312 = global read "Global.vi" "程序固化引用句柄"() -> (w362:refnum<vi>)
                    n313 = property class="检测CTR"(reference=w362, "Value"=T4."Runing" ("值")) -> ()  [unwired: 1 in, 2 out]
                    n314 = call "设备状态.vi"("枚举"=enum16{"Read", "Write"}."Write", "工位"=enum16{"工位一", "工位二"}."工位二", "Status_Write"=i16 200) -> ()  [unwired: 8 in, 1 out]
                  }
                  frame #1 {
                    n315 = Wait (ms)(milliseconds to wait=u32 500 ("等待时间（毫秒）")) -> ()  [unwired: 1 out]
                  }
                  frame #2 {
                    n316 = local read "SENSOR"() -> (w368:T1)
                    n317 = call "FirmwareProgramming2.vi"("SENSOR"=w368) -> ("Message"=w366:string, "Done?"=w367:bool)  [unwired: 8 in, 1 out]
                    n318 = case shown="真" w367 {
                      tunnel: w366 -> [w377 _]
                      tunnel: ["不合格" "报表"] -> w365
                      frame False {
                        n319 = global read "Global.vi" "程序固化引用句柄"() -> (w379:refnum<vi>)
                        n320 = call "设备状态.vi"("枚举"=enum16{"Read", "Write"}."Write", "工位"=enum16{"工位一", "工位二"}."工位二", "Status_Write"=i16 400) -> ()  [unwired: 8 in, 1 out]
                        n321 = local read "判定结果"() -> (w372:bool[][])
                        n322 = Build Array (concatenate)(w372, bool[][] [[TRUE, FALSE]] ("判定结果")) -> (w374:bool[][])
                        n323 = Concatenate Strings("程序固化失败！\n可能的原因是：\n" ("字符串"), w377) -> (w376:string)
                        n324 = property class="检测CTR"(reference=w379, "Value"=T4."Faild" ("值")) -> ()  [unwired: 1 in, 2 out]
                        n325 = local write "判定结果"(w374) -> ()
                        n326 = One Button Dialog(message=w376) -> ()  [unwired: 1 in, 1 out]
                      }
                      frame True {
                        n327 = local read "判定结果"() -> (w384:bool[][])
                        n328 = global read "Global.vi" "程序固化引用句柄"() -> (w388:refnum<vi>)
                        n329 = Build Array (concatenate)(w384, bool[][] [[TRUE, TRUE]] ("判定结果")) -> (w386:bool[][])
                        n330 = local write "判定结果"(w386) -> ()
                        n331 = property class="检测CTR"(reference=w388, "Value"=T4."Pass" ("值")) -> ()  [unwired: 1 in, 2 out]
                        n332 = call "设备状态.vi"("枚举"=enum16{"Read", "Write"}."Write", "工位"=enum16{"工位一", "工位二"}."工位二", "Status_Write"=i16 400) -> ()  [unwired: 8 in, 1 out]
                      }
                    }
                    n333 = local write "STEP"(w365) -> ()
                  }
                }
              }
              frame True {
                n334 = call "设备状态.vi"("枚举"=enum16{"Read", "Write"}."Write", "工位"=enum16{"工位一", "工位二"}."工位二", "Status_Write"=i16 400) -> ()  [unwired: 8 in, 1 out]
                n335 = local read "判定结果"() -> (w394:bool[][])
                n336 = local write "STEP"("报表" ("STEP")) -> ()
                n337 = Build Array (concatenate)(w394, bool[][] [[FALSE, FALSE]] ("判定结果")) -> (w396:bool[][])
                n338 = local write "判定结果"(w396) -> ()
              }
            }
          }
          frame "程序复检" {
            n339 = global read "Global.vi" "传感器特性用句柄"() -> (w401:refnum<vi>)
            n340 = property class="检测CTR"(reference=w401) -> ("Value"=w402:variant)  [unwired: 1 in, 2 out]
            n341 = Variant To Data(type=检测CTR数据."Idle" ("Data"), Variant=w402) -> (data=w400:T2)  [unwired: 1 in, 1 out]
            n342 = Equal?(x=w400, y=检测CTR数据."Skip" ("Data")) -> (x = y?=w397:bool)
            n343 = case shown="假" w397 {
              frame False {
                n344 = stacked-sequence {
                  frame #0 {
                    n345 = global read "Global.vi" "传感器特性用句柄"() -> (w404:refnum<vi>)
                    n346 = call "浮动通知.vi"("通知内容"="传感器特性" ("Status")) -> ()  [unwired: 11 in]
                    n347 = property class="检测CTR"(reference=w404, "Value"=T4."Runing" ("值")) -> ()  [unwired: 1 in, 2 out]
                  }
                  frame #1 {
                    n348 = vi-ref "T1T2占空比.vi"() -> (w407:refnum<vi>)
                    n349 = call "CallVI.vi"("VI引用"=w407, "状态"=T3."Hidden") -> ()  [unwired: 12 in, 2 out]
                    n350 = local write "STEP"("自动" ("STEP")) -> ()
                    n351 = call "设备状态.vi"("枚举"=enum16{"Read", "Write"}."Write", "工位"=enum16{"工位一", "工位二"}."工位二", "Status_Write"=i16 300) -> ()  [unwired: 8 in, 1 out]
                  }
                  frame #2 {
                    n352 = vi-ref "扭矩.vi"() -> (w413:refnum<vi>)
                    n353 = call "CallVI.vi"("VI引用"=w413, "状态"=T3."Hidden") -> ()  [unwired: 12 in, 2 out]
                  }
                }
              }
              frame True {
                n354 = local read "判定结果"() -> (w414:bool[][])
                n355 = local write "STEP"("程序固化" ("STEP")) -> ()
                n356 = Build Array (concatenate)(w414, bool[][] [[FALSE, FALSE]] ("判定结果")) -> (w416:bool[][])
                n357 = local write "判定结果"(w416) -> ()
              }
            }
          }
          frame "复检判定" {
            n358 = global read "Global.vi" "复检判定参数"() -> (w429:T8)
            n359 = local read "传感器特性"() -> (w430:cluster{dbl[], dbl[]}[])
            n360 = global read "Global.vi" "Result"() -> (w431:refnum<vi>)
            n361 = global read "Global.vi" "传感器特性用句柄"() -> (w428:refnum<vi>)
            n362 = call "对中台复检判定.vi"("Result"=w431, "判定参数"=w429, "XY曲线"=w430) -> ("OK？"=w419:bool)  [unwired: 8 in]
            n363 = call "CloseVI.vi"("名称或相对路径"="T1T2占空比.vi") -> ()  [unwired: 10 in, 1 out]
            n364 = Select(t=T4."Pass" ("值"), s=w419, f=T4."Faild" ("值")) -> (s? t:f=w425:T4)
            n365 = Build Array(TRUE ("元素"), w419) -> (w421:bool[])
            n366 = local read "判定结果"() -> (w423:bool[][])
            n367 = property class="检测CTR"(reference=w428, "Value"=w425) -> ()  [unwired: 1 in, 2 out]
            n368 = case shown="真" w419 {
              selector: w419 -> [w442 w450]
              frame False {
                w445 = enum16{"Read", "Write"}."Write" ("枚举")
                n369 = call "设备状态.vi"("枚举"=w445, "工位"=enum16{"工位一", "工位二"}."工位二", "Status_Write"=i16 400) -> ()  [unwired: 8 in, 1 out]
                n370 = local write "合格状态"(w442) -> ()
                n371 = local write "STEP"("报表" ("STEP")) -> ()
                n372 = call "合格状态.vi"("枚举"=w445, "工位"=enum16{"工位一", "工位二"}."工位二", "Status_Write"=i16 2) -> ()  [unwired: 8 in, 1 out]
              }
              frame True {
                n373 = local write "STEP"("程序固化" ("STEP")) -> ()
                "合格状态" <- w450
              }
            }
            n374 = Build Array(w421) -> (w420:bool[][])
            n375 = Build Array (concatenate)(w423, w420) -> (w424:bool[][])
            n376 = local write "判定结果"(w424) -> ()
            n377 = disable-structure shown="禁用" {
              frame Disabled {
                n378 = Two Button Dialog(message="复检失败\n请选择是否继续？" ("消息"), 1:"否" ("F按钮名称（“取消”）"), 2:"是" ("T按钮名称（“确定”）")) -> (T button?=w435:bool)
                n379 = case shown="假" w435 {
                  tunnel: ["报表" ("STEP") "程序固化" ("STEP")] -> w436
                  frame False {
                    n380 = call "设备状态.vi"("枚举"=enum16{"Read", "Write"}."Write", "工位"=enum16{"工位一", "工位二"}."工位一", "Status_Write"=i16 400) -> ()  [unwired: 8 in, 1 out]
                  }
                  frame True {
                  }
                }
                n381 = local write "STEP"(w436) -> ()
              }
              frame Enabled {
              }
            }
          }
          frame "自动" {
            n382 = global read "Global.vi" "产品型号"() -> (w451:string)
            n383 = call "设备状态.vi"("工位"=enum16{"工位一", "工位二"}."工位二") -> ("Status_Read"=w453:i16)  [unwired: 10 in]
            n384 = case shown="10" w453 {
              tunnel: w451 -> [_ _ _ _ _ w461 _ _ _ _ _ _ _ _ _ _ _ _ _ _ _ _ _ _ _ _ _ _ _]
              frame -128 {
                n385 = call "浮动通知.vi"("通知内容"="复位中……" ("Status")) -> ()  [unwired: 11 in]
                n386 = global write "Global.vi" "计时开始"(FALSE ("计时开始")) -> ()
              }
              frame 0, Default {
              }
              frame 1 {
                n387 = call "浮动通知.vi"("通知内容"="请复位！" ("Status")) -> ()  [unwired: 11 in]
              }
              frame 5 {
                n388 = global write "Global.vi" "计时开始"(FALSE ("计时开始")) -> ()
                n389 = call "浮动通知.vi"("通知内容"="复位完成" ("Status")) -> ()  [unwired: 11 in]
              }
              frame 8 {
                n390 = call "浮动通知.vi"("通知内容"="程序停止！" ("Status")) -> ()  [unwired: 11 in]
              }
              frame 10 {
                n391 = Wait Until Next ms Multiple(millisecond multiple=u32 50 ("等待时间（毫秒）")) -> ()  [unwired: 1 out]
                n392 = case shown="\"R563X\"" w461 {
                  tunnel: [_ "扫码" ("STEP") "扫码" ("STEP") "传感器码" ("STEP") "传感器码" ("STEP") "传感器码" ("STEP") "传感器码" ("STEP") "传感器码" ("STEP")] -> w460
                  frame "假", Default {
                  }
                  frame "R128" {
                  }
                  frame "R567X" {
                  }
                  frame "R128K" {
                  }
                  frame "R128G" {
                  }
                  frame "R128H" {
                  }
                  frame "R092B" {
                  }
                  frame "R563X" {
                  }
                }
                n393 = local write "STEP"(w460) -> ()
              }
              frame 300 {
                n394 = call "设备状态.vi"("枚举"=enum16{"Read", "Write"}."Write", "工位"=enum16{"工位一", "工位二"}."工位二", "Status_Write"=i16 310) -> ()  [unwired: 8 in, 1 out]
              }
              frame 310 {
                n395 = call "传感器数据.vi"() -> ("传感器读数"=w477:T6)  [unwired: 11 in]
                n396 = global read "excursion.vi" "excursion"() -> (w475:T7)
                n397 = global read "Global.vi" "工位二扭矩"() -> (w473:dbl)
                n398 = global read "Global.vi" "扭矩"() -> (w487:cluster{"工位一":dbl, "工位二":dbl})
                n399 = Unbundle By Name(w477) -> ("工位二驱动伺服位移"=w478:sgl)
                n400 = Unbundle By Name(w487) -> ()  [unwired: 1 out]
                n401 = global read "Global.vi" "保护角度"() -> (w482:dbl)
                n402 = Unbundle By Name(w475) -> ("左上升"=w474:dbl)
                n403 = local read "初始角度"() -> (w479:dbl)
                n404 = Subtract(x=w478, y=w479) -> (x-y=w480:dbl)
                n405 = Subtract(x=w473, y=w474) -> (x-y=w485:dbl)
                n406 = Absolute Value(x=w480) -> (abs(x)=w481:dbl)
                n407 = Less Or Equal?(x=w485, y=-6.0) -> (x <= y?=w484:bool)
                n408 = Greater Or Equal?(x=w481, y=w482) -> (x >= y?=w476:bool)
                n409 = Compound Arithmetic op=OR ("复合运算")(w484, w476) -> (w483:bool)
                n410 = case shown="真" w483 {
                  tunnel: w473 -> [w489 _]
                  tunnel: w476 -> [_ w512]
                  frame False {
                    n411 = feedback #1() -> (w505:dbl)  [unwired: 1 in]
                    n412 = feedback-in #1(w489) -> ()
                    n413 = feedback #2() -> (w497:dbl)  [unwired: 1 in]
                    n414 = Equal?(x=w489, y=w505) -> (x = y?=w503:bool)
                    n415 = feedback #3() -> (w504:dbl)  [unwired: 1 in]
                    n416 = feedback-in #3(w505) -> ()
                    n417 = feedback #4() -> (w496:dbl)  [unwired: 1 in]
                    n418 = feedback-in #4(w497) -> ()
                    n419 = Equal?(x=w489, y=w497) -> (x = y?=w494:bool)
                    n420 = feedback #5() -> (w495:dbl)  [unwired: 1 in]
                    n421 = feedback-in #5(w496) -> ()
                    n422 = Equal?(x=w489, y=w504) -> (x = y?=w502:bool)
                    n423 = Equal?(x=w489, y=w496) -> (x = y?=w493:bool)
                    n424 = feedback #6() -> (w500:dbl)  [unwired: 1 in]
                    n425 = feedback-in #6(w504) -> ()
                    n426 = feedback #7() -> (w490:dbl)  [unwired: 1 in]
                    n427 = feedback-in #7(w495) -> ()
                    n428 = Equal?(x=w489, y=w500) -> (x = y?=w501:bool)
                    n429 = feedback #8() -> (w498:dbl)  [unwired: 1 in]
                    n430 = feedback-in #2(w498) -> ()
                    n431 = feedback-in #8(w500) -> ()
                    n432 = Equal?(x=w489, y=w495) -> (x = y?=w492:bool)
                    n433 = Equal?(x=w489, y=w498) -> (x = y?=w499:bool)
                    n434 = Equal?(x=w489, y=w490) -> (x = y?=w491:bool)
                    n435 = Compound Arithmetic op=AND(w503, w502, w501, w499, w494, w493, w492, w491) -> ()  [unwired: 1 out]
                    n436 = case shown="真" FALSE {
                      frame False {
                      }
                      frame True {
                        n437 = call "设备状态.vi"("枚举"=enum16{"Read", "Write"}."Write", "工位"=enum16{"工位一", "工位二"}."工位二", "Status_Write"=i16 316) -> ()  [unwired: 8 in, 1 out]
                        n438 = One Button Dialog(message="扭矩采集异常！\n请重启应用程序！" ("消息")) -> (true=w509:bool)  [unwired: 1 in]
                        n439 = case shown="假" w509 {
                          frame False {
                            n440 = local write "STEP"("报表") -> ()
                          }
                          frame True {
                          }
                        }
                      }
                    }
                  }
                  frame True {
                    n441 = case shown="真" w512 {
                      frame False {
                        n442 = call "设备状态.vi"("枚举"=enum16{"Read", "Write"}."Write", "工位"=enum16{"工位一", "工位二"}."工位二", "Status_Write"=i16 311) -> ()  [unwired: 8 in, 1 out]
                      }
                      frame True {
                        n443 = call "设备状态.vi"("枚举"=enum16{"Read", "Write"}."Write", "工位"=enum16{"工位一", "工位二"}."工位二", "Status_Write"=i16 316) -> ()  [unwired: 8 in, 1 out]
                        n444 = One Button Dialog(message="扭矩采集异常！\n请重启应用程序！" ("消息")) -> (true=w519:bool)  [unwired: 1 in]
                        n445 = case shown="真" w519 {
                          frame False {
                          }
                          frame True {
                            n446 = local write "STEP"("报表" ("STEP")) -> ()
                          }
                        }
                      }
                    }
                  }
                }
              }
              frame 311 {
                n447 = global read "Global.vi" "扭矩"() -> (w527:cluster{"工位一":dbl, "工位二":dbl})
                n448 = global read "excursion.vi" "excursion"() -> (w524:T7)
                n449 = global read "Global.vi" "工位二扭矩"() -> (w522:dbl)
                n450 = Unbundle By Name(w527) -> ()  [unwired: 1 out]
                n451 = Unbundle By Name(w524) -> ("左下降"=w523:dbl)
                n452 = Subtract(x=w522, y=w523) -> (x-y=w526:dbl)
                n453 = Greater Or Equal To 0?(x=w526) -> (x >= 0?=w525:bool)
                n454 = case shown="真" w525 {
                  frame False {
                  }
                  frame True {
                    n455 = flat-sequence {
                      frame #0 {
                        n456 = call "设备状态.vi"("枚举"=enum16{"Read", "Write"}."Write", "工位"=enum16{"工位一", "工位二"}."工位二", "Status_Write"=i16 312) -> ()  [unwired: 8 in, 1 out]
                        n457 = call "工位暂停.vi"("枚举"=enum16{"Read", "Write"}."Write", "工位"=enum16{"工位一", "工位二"}."工位二", "Status_Write"=i16 1) -> ()  [unwired: 8 in, 1 out]
                      }
                      frame #1 {
                        n458 = Wait (ms)(milliseconds to wait=u32 500 ("等待时间（毫秒）")) -> ()  [unwired: 1 out]
                      }
                    }
                  }
                }
              }
              frame 312 {
                n459 = call "传感器数据.vi"() -> ("传感器读数"=w539:T6)  [unwired: 11 in]
                n460 = global read "excursion.vi" "excursion"() -> (w538:T7)
                n461 = global read "Global.vi" "扭矩"() -> (w550:cluster{"工位一":dbl, "工位二":dbl})
                n462 = Unbundle By Name(w539) -> ("工位二驱动伺服位移"=w540:sgl)
                n463 = global read "Global.vi" "工位二扭矩"() -> (w536:dbl)
                n464 = global read "Global.vi" "保护角度"() -> (w544:dbl)
                n465 = Unbundle By Name(w550) -> ()  [unwired: 1 out]
                n466 = local read "初始角度"() -> (w541:dbl)
                n467 = global read "Global.vi" "复检参数"() -> (w549:T9)
                n468 = Unbundle By Name(w538) -> ("右上升"=w537:dbl)
                n469 = Subtract(x=w540, y=w541) -> (x-y=w542:dbl)
                n470 = Unbundle By Name(w549) -> ("换向扭矩"=w548:dbl)
                n471 = Subtract(x=w536, y=w537) -> (x-y=w546:dbl)
                n472 = Absolute Value(x=w542) -> (abs(x)=w543:dbl)
                n473 = Greater Or Equal?(x=w543, y=w544) -> (x >= y?=w535:bool)
                n474 = Greater Or Equal?(x=w546, y=w548) -> (x >= y?=w547:bool)
                n475 = Compound Arithmetic op=OR ("复合运算")(w547, w535) -> (w545:bool)
                n476 = case shown="假" w545 {
                  tunnel: w546 -> [w553 _]
                  tunnel: w535 -> [_ w616]
                  frame False {
                    n477 = Greater Or Equal?(x=w553, y=0.0) -> (x >= y?=w551:bool)
                    n478 = case shown="真" w551 {
                      tunnel: w553 -> [_ w559]
                      frame False {
                      }
                      frame True {
                        n479 = local read "传感器特性"() -> (w560:cluster{dbl[], dbl[]}[])
                        n480 = local read "初始化"() -> (w558:bool[])
                        n481 = for "For循环" {
                          tunnel: w560 -> [w568] mode=indexing
                          tunnel: [w567] -> w561 mode=indexing
                          tunnel: w559 -> [w566]
                          tunnel: w558 -> [w565] mode=indexing
                          tunnel: [w564] -> w557 mode=indexing
                          i -> [w569]
                          n482 = case shown="0" w569 {
                            tunnel: w568 -> [w571 w582 w596 w612]
                            tunnel: [w571 w580 w594 w608] -> w567
                            tunnel: w566 -> [_ w578 w591 w605]
                            tunnel: w565 -> [w570 w573 w588 w603]
                            tunnel: [w570 FALSE ("布尔") FALSE ("布尔") FALSE ("布尔")] -> w564
                            tunnel: 2 -> [_ w572 w587 w600]
                            tunnel: 2 -> [_ w576 w590 w604]
                            frame Default {
                            }
                            frame 0 {
                              n483 = global read "Global.vi" "工位二T1"() -> (w575:dbl)
                              n484 = Unbundle(w582) -> (w585:dbl[], w581:dbl[])
                              n485 = call-poly <userlib>:"MGI Running Average.vi"("Averaging Size"=w576, "Initialize? (F)"=w573, "Value"=w578) -> ("Average"=w577:dbl)  [unwired: 8 in]
                              n486 = call-poly <userlib>:"MGI Running Average.vi"("Averaging Size"=w572, "Initialize? (F)"=w573, "Value"=w575) -> ("Average"=w574:dbl)  [unwired: 8 in]
                              n487 = Build Array (concatenate)(w585, w577) -> (w584:dbl[])
                              n488 = Build Array (concatenate)(w581, w574) -> (w583:dbl[])
                              n489 = Bundle(w584, w583) -> (w580:cluster{dbl[], dbl[]})  [unwired: 1 in]
                            }
                            frame 1 {
                              n490 = Unbundle(w596) -> (w599:dbl[], w595:dbl[])
                              n491 = global read "Global.vi" "工位二T2"() -> (w589:dbl)
                              n492 = call-poly <userlib>:"MGI Running Average.vi"("Averaging Size"=w590, "Initialize? (F)"=w588, "Value"=w591) -> ("Average"=w592:dbl)  [unwired: 8 in]
                              n493 = call-poly <userlib>:"MGI Running Average.vi"("Averaging Size"=w587, "Initialize? (F)"=w588, "Value"=w589) -> ("Average"=w586:dbl)  [unwired: 8 in]
                              n494 = Build Array (concatenate)(w599, w592) -> (w598:dbl[])
                              n495 = Build Array (concatenate)(w595, w586) -> (w597:dbl[])
                              n496 = Bundle(w598, w597) -> (w594:cluster{dbl[], dbl[]})  [unwired: 1 in]
                            }
                            frame 2 {
                              n497 = Unbundle(w612) -> (w615:dbl[], w611:dbl[])
                              n498 = global read "Global.vi" "工位二T1"() -> (w610:dbl)
                              n499 = global read "Global.vi" "工位二T2"() -> (w609:dbl)
                              n500 = call-poly <userlib>:"MGI Running Average.vi"("Averaging Size"=w604, "Initialize? (F)"=w603, "Value"=w605) -> ("Average"=w606:dbl)  [unwired: 8 in]
                              n501 = Add(x=w610, y=w609) -> (x+y=w602:dbl)
                              n502 = call-poly <userlib>:"MGI Running Average.vi"("Averaging Size"=w600, "Initialize? (F)"=w603, "Value"=w602) -> ("Average"=w601:dbl)  [unwired: 8 in]
                              n503 = Build Array (concatenate)(w615, w606) -> (w614:dbl[])
                              n504 = Build Array (concatenate)(w611, w601) -> (w613:dbl[])
                              n505 = Bundle(w614, w613) -> (w608:cluster{dbl[], dbl[]})  [unwired: 1 in]
                            }
                          }
                        }
                        n506 = local write "初始化"(w557) -> ()
                        n507 = local write "传感器特性"(w561) -> ()
                      }
                    }
                    n508 = call "工位暂停.vi"("枚举"=enum16{"Read", "Write"}."Write", "工位"=enum16{"工位一", "工位二"}."工位二", "Status_Write"=i16 0) -> ()  [unwired: 8 in, 1 out]
                  }
                  frame True {
                    n509 = case shown="假" w616 {
                      frame False {
                        n510 = call "工位暂停.vi"("枚举"=enum16{"Read", "Write"}."Write", "工位"=enum16{"工位一", "工位二"}."工位二", "Status_Write"=i16 1) -> ()  [unwired: 8 in, 1 out]
                        n511 = call "设备状态.vi"("枚举"=enum16{"Read", "Write"}."Write", "工位"=enum16{"工位一", "工位二"}."工位二", "Status_Write"=i16 313) -> ()  [unwired: 8 in, 1 out]
                      }
                      frame True {
                        n512 = call "设备状态.vi"("枚举"=enum16{"Read", "Write"}."Write", "工位"=enum16{"工位一", "工位二"}."工位二", "Status_Write"=i16 316) -> ()  [unwired: 8 in, 1 out]
                        n513 = One Button Dialog(message="扭矩采集异常！\n请重启应用程序！" ("消息")) -> (true=w626:bool)  [unwired: 1 in]
                        n514 = case shown="假" w626 {
                          frame False {
                            n515 = local write "STEP"("报表" ("STEP")) -> ()
                          }
                          frame True {
                          }
                        }
                      }
                    }
                  }
                }
              }
              frame 313 {
                n516 = global read "excursion.vi" "excursion"() -> (w631:T7)
                n517 = global read "Global.vi" "扭矩"() -> (w637:cluster{"工位一":dbl, "工位二":dbl})
                n518 = global read "Global.vi" "工位二扭矩"() -> (w629:dbl)
                n519 = Unbundle By Name(w637) -> ()  [unwired: 1 out]
                n520 = global read "Global.vi" "复检参数"() -> (w635:T9)
                n521 = Unbundle By Name(w631) -> ("右下降"=w630:dbl)
                n522 = Unbundle By Name(w635) -> ("换向扭矩"=w633:dbl)
                n523 = Subtract(x=w629, y=w630) -> (x-y=w634:dbl)
                n524 = Less Than 0?(x=w634) -> (x < 0?=w636:bool)
                n525 = Less Or Equal?(x=w634, y=w633) -> (x <= y?=w632:bool)
                n526 = case shown="假" w636 {
                  tunnel: w634 -> [w639 _]
                  tunnel: w632 -> [w638 _]
                  frame False {
                    n527 = case shown="真" w638 {
                      tunnel: w639 -> [_ w645]
                      frame False {
                      }
                      frame True {
                        n528 = local read "传感器特性"() -> (w646:cluster{dbl[], dbl[]}[])
                        n529 = local read "初始化"() -> (w644:bool[])
                        n530 = for "For循环" {
                          tunnel: w646 -> [w654] mode=indexing
                          tunnel: [w653] -> w647 mode=indexing
                          tunnel: w645 -> [w652]
                          tunnel: w644 -> [w651] mode=indexing
                          tunnel: [w650] -> w643 mode=indexing
                          i -> [w655]
                          n531 = case shown="5" w655 {
                            tunnel: w654 -> [w657 w668 w682 w698]
                            tunnel: [w657 w666 w680 w694] -> w653
                            tunnel: w652 -> [_ w664 w678 w692]
                            tunnel: w651 -> [w656 w660 w672 w688]
                            tunnel: [w656 FALSE ("布尔") FALSE ("布尔") FALSE ("布尔")] -> w650
                            tunnel: 2 -> [_ w659 w673 w687]
                            tunnel: 2 -> [_ w662 w676 w690]
                            frame Default {
                            }
                            frame 3 {
                              n532 = Unbundle(w668) -> (w671:dbl[], w667:dbl[])
                              n533 = global read "Global.vi" "工位二T1"() -> (w661:dbl)
                              n534 = call-poly <userlib>:"MGI Running Average.vi"("Averaging Size"=w662, "Initialize? (F)"=w660, "Value"=w664) -> ("Average"=w663:dbl)  [unwired: 8 in]
                              n535 = call-poly <userlib>:"MGI Running Average.vi"("Averaging Size"=w659, "Initialize? (F)"=w660, "Value"=w661) -> ("Average"=w658:dbl)  [unwired: 8 in]
                              n536 = Build Array (concatenate)(w671, w663) -> (w670:dbl[])
                              n537 = Build Array (concatenate)(w667, w658) -> (w669:dbl[])
                              n538 = Bundle(w670, w669) -> (w666:cluster{dbl[], dbl[]})  [unwired: 1 in]
                            }
                            frame 4 {
                              n539 = Unbundle(w682) -> (w685:dbl[], w681:dbl[])
                              n540 = global read "Global.vi" "工位二T2"() -> (w675:dbl)
                              n541 = call-poly <userlib>:"MGI Running Average.vi"("Averaging Size"=w676, "Initialize? (F)"=w672, "Value"=w678) -> ("Average"=w677:dbl)  [unwired: 8 in]
                              n542 = call-poly <userlib>:"MGI Running Average.vi"("Averaging Size"=w673, "Initialize? (F)"=w672, "Value"=w675) -> ("Average"=w674:dbl)  [unwired: 8 in]
                              n543 = Build Array (concatenate)(w681, w674) -> (w683:dbl[])
                              n544 = Build Array (concatenate)(w685, w677) -> (w684:dbl[])
                              n545 = Bundle(w684, w683) -> (w680:cluster{dbl[], dbl[]})  [unwired: 1 in]
                            }
                            frame 5 {
                              n546 = Unbundle(w698) -> (w701:dbl[], w697:dbl[])
                              n547 = global read "Global.vi" "工位二T1"() -> (w696:dbl)
                              n548 = global read "Global.vi" "工位二T2"() -> (w695:dbl)
                              n549 = call-poly <userlib>:"MGI Running Average.vi"("Averaging Size"=w690, "Initialize? (F)"=w688, "Value"=w692) -> ("Average"=w691:dbl)  [unwired: 8 in]
                              n550 = Add(x=w696, y=w695) -> (x+y=w689:dbl)
                              n551 = call-poly <userlib>:"MGI Running Average.vi"("Averaging Size"=w687, "Initialize? (F)"=w688, "Value"=w689) -> ("Average"=w686:dbl)  [unwired: 8 in]
                              n552 = Build Array (concatenate)(w701, w691) -> (w700:dbl[])
                              n553 = Build Array (concatenate)(w697, w686) -> (w699:dbl[])
                              n554 = Bundle(w700, w699) -> (w694:cluster{dbl[], dbl[]})  [unwired: 1 in]
                            }
                          }
                        }
                        n555 = call "工位暂停.vi"("枚举"=enum16{"Read", "Write"}."Write", "工位"=enum16{"工位一", "工位二"}."工位二", "Status_Write"=i16 0) -> ()  [unwired: 8 in, 1 out]
                        n556 = local write "初始化"(w643) -> ()
                        n557 = local write "传感器特性"(w647) -> ()
                      }
                    }
                  }
                  frame True {
                    n558 = flat-sequence {
                      frame #0 {
                        n559 = call "设备状态.vi"("枚举"=enum16{"Read", "Write"}."Write", "工位"=enum16{"工位一", "工位二"}."工位二", "Status_Write"=i16 314) -> ()  [unwired: 8 in, 1 out]
                        n560 = call "工位暂停.vi"("枚举"=enum16{"Read", "Write"}."Write", "工位"=enum16{"工位一", "工位二"}."工位二", "Status_Write"=i16 1) -> ()  [unwired: 8 in, 1 out]
                      }
                      frame #1 {
                        n561 = Wait (ms)(milliseconds to wait=u32 500 ("等待时间（毫秒）")) -> ()  [unwired: 1 out]
                      }
                    }
                  }
                }
              }
              frame 314 {
                n562 = call "传感器数据.vi"() -> ("传感器读数"=w714:T6)  [unwired: 11 in]
                n563 = global read "Global.vi" "复检参数"() -> (w723:T9)
                n564 = global read "Global.vi" "扭矩"() -> (w724:cluster{"工位一":dbl, "工位二":dbl})
                n565 = global read "Global.vi" "工位二扭矩"() -> (w709:dbl)
                n566 = global read "excursion.vi" "excursion"() -> (w711:T7)
                n567 = Unbundle By Name(w714) -> ("工位二驱动伺服位移"=w715:sgl)
                n568 = global read "Global.vi" "保护角度"() -> (w719:dbl)
                n569 = Unbundle By Name(w724) -> ()  [unwired: 1 out]
                n570 = Unbundle By Name(w723) -> ("换向扭矩"=w722:dbl)
                n571 = local read "初始角度"() -> (w716:dbl)
                n572 = Unbundle By Name(w711) -> ("左上升"=w710:dbl)
                n573 = Subtract(x=w715, y=w716) -> (x-y=w717:dbl)
                n574 = Negate(x=w722) -> (-x=w725:dbl)
                n575 = Subtract(x=w709, y=w710) -> (x-y=w720:dbl)
                n576 = Absolute Value(x=w717) -> (abs(x)=w718:dbl)
                n577 = Less Or Equal?(x=w720, y=w725) -> (x <= y?=w721:bool)
                n578 = Greater Or Equal?(x=w718, y=w719) -> (x >= y?=w712:bool)
                n579 = Compound Arithmetic op=OR ("复合运算")(w721, w712) -> (w713:bool)
                n580 = case shown="假" w713 {
                  tunnel: w720 -> [w731 _]
                  tunnel: w720 -> [w729 _]
                  tunnel: w712 -> [_ w791]
                  frame False {
                    n581 = Less Or Equal To 0?(x=w729) -> (x <= 0?=w730:bool)
                    n582 = case shown="真" w730 {
                      tunnel: w731 -> [_ w734]
                      frame False {
                      }
                      frame True {
                        n583 = local read "传感器特性"() -> (w735:cluster{dbl[], dbl[]}[])
                        n584 = local read "初始化"() -> (w733:bool[])
                        n585 = for "For循环" {
                          tunnel: w735 -> [w743] mode=indexing
                          tunnel: [w742] -> w736 mode=indexing
                          tunnel: w734 -> [w741]
                          tunnel: w733 -> [w740] mode=indexing
                          tunnel: [w739] -> w732 mode=indexing
                          i -> [w744]
                          n586 = case shown="6" w744 {
                            tunnel: w743 -> [w746 w757 w771 w787]
                            tunnel: [w746 w755 w769 w783] -> w742
                            tunnel: w741 -> [_ w752 w767 w781]
                            tunnel: w740 -> [w745 w749 w763 w775]
                            tunnel: [w745 FALSE ("布尔") FALSE ("布尔") FALSE ("布尔")] -> w739
                            tunnel: 2 -> [_ w748 w762 w776]
                            tunnel: 2 -> [_ w751 w765 w779]
                            frame Default {
                            }
                            frame 6 {
                              n587 = Unbundle(w757) -> (w760:dbl[], w756:dbl[])
                              n588 = global read "Global.vi" "工位二T1"() -> (w750:dbl)
                              n589 = call-poly <userlib>:"MGI Running Average.vi"("Averaging Size"=w751, "Initialize? (F)"=w749, "Value"=w752) -> ("Average"=w753:dbl)  [unwired: 8 in]
                              n590 = call-poly <userlib>:"MGI Running Average.vi"("Averaging Size"=w748, "Initialize? (F)"=w749, "Value"=w750) -> ("Average"=w747:dbl)  [unwired: 8 in]
                              n591 = Build Array (concatenate)(w760, w753) -> (w759:dbl[])
                              n592 = Build Array (concatenate)(w756, w747) -> (w758:dbl[])
                              n593 = Bundle(w759, w758) -> (w755:cluster{dbl[], dbl[]})  [unwired: 1 in]
                            }
                            frame 7 {
                              n594 = Unbundle(w771) -> (w774:dbl[], w770:dbl[])
                              n595 = global read "Global.vi" "工位二T2"() -> (w764:dbl)
                              n596 = call-poly <userlib>:"MGI Running Average.vi"("Averaging Size"=w765, "Initialize? (F)"=w763, "Value"=w767) -> ("Average"=w766:dbl)  [unwired: 8 in]
                              n597 = call-poly <userlib>:"MGI Running Average.vi"("Averaging Size"=w762, "Initialize? (F)"=w763, "Value"=w764) -> ("Average"=w761:dbl)  [unwired: 8 in]
                              n598 = Build Array (concatenate)(w770, w761) -> (w772:dbl[])
                              n599 = Build Array (concatenate)(w774, w766) -> (w773:dbl[])
                              n600 = Bundle(w773, w772) -> (w769:cluster{dbl[], dbl[]})  [unwired: 1 in]
                            }
                            frame 8 {
                              n601 = Unbundle(w787) -> (w790:dbl[], w786:dbl[])
                              n602 = global read "Global.vi" "工位二T1"() -> (w785:dbl)
                              n603 = global read "Global.vi" "工位二T2"() -> (w784:dbl)
                              n604 = call-poly <userlib>:"MGI Running Average.vi"("Averaging Size"=w779, "Initialize? (F)"=w775, "Value"=w781) -> ("Average"=w780:dbl)  [unwired: 8 in]
                              n605 = Add(x=w785, y=w784) -> (x+y=w778:dbl)
                              n606 = call-poly <userlib>:"MGI Running Average.vi"("Averaging Size"=w776, "Initialize? (F)"=w775, "Value"=w778) -> ("Average"=w777:dbl)  [unwired: 8 in]
                              n607 = Build Array (concatenate)(w790, w780) -> (w789:dbl[])
                              n608 = Build Array (concatenate)(w786, w777) -> (w788:dbl[])
                              n609 = Bundle(w789, w788) -> (w783:cluster{dbl[], dbl[]})  [unwired: 1 in]
                            }
                          }
                        }
                        n610 = local write "初始化"(w732) -> ()
                        n611 = local write "传感器特性"(w736) -> ()
                      }
                    }
                    n612 = call "工位暂停.vi"("枚举"=enum16{"Read", "Write"}."Write", "工位"=enum16{"工位一", "工位二"}."工位二", "Status_Write"=i16 0) -> ()  [unwired: 8 in, 1 out]
                  }
                  frame True {
                    n613 = case shown="假" w791 {
                      frame False {
                        n614 = call "设备状态.vi"("枚举"=enum16{"Read", "Write"}."Write", "工位"=enum16{"工位一", "工位二"}."工位二", "Status_Write"=i16 315) -> ()  [unwired: 8 in, 1 out]
                        n615 = call "工位暂停.vi"("枚举"=enum16{"Read", "Write"}."Write", "工位"=enum16{"工位一", "工位二"}."工位二", "Status_Write"=i16 1) -> ()  [unwired: 8 in, 1 out]
                      }
                      frame True {
                        n616 = call "设备状态.vi"("枚举"=enum16{"Read", "Write"}."Write", "工位"=enum16{"工位一", "工位二"}."工位二", "Status_Write"=i16 316) -> ()  [unwired: 8 in, 1 out]
                        n617 = One Button Dialog(message="扭矩采集异常！\n请重启应用程序！" ("消息")) -> (true=w801:bool)  [unwired: 1 in]
                        n618 = case shown="假" w801 {
                          frame False {
                            n619 = local write "STEP"("报表" ("STEP")) -> ()
                          }
                          frame True {
                          }
                        }
                      }
                    }
                  }
                }
              }
              frame 315 {
                n620 = global read "Global.vi" "复检参数"() -> (w810:T9)
                n621 = global read "Global.vi" "扭矩"() -> (w813:cluster{"工位一":dbl, "工位二":dbl})
                n622 = global read "excursion.vi" "excursion"() -> (w806:T7)
                n623 = global read "Global.vi" "工位二扭矩"() -> (w804:dbl)
                n624 = Unbundle By Name(w813) -> ()  [unwired: 1 out]
                n625 = Unbundle By Name(w810) -> ("换向扭矩"=w809:dbl)
                n626 = Unbundle By Name(w806) -> ("左下降"=w805:dbl)
                n627 = Negate(x=w809) -> (-x=w808:dbl)
                n628 = Subtract(x=w804, y=w805) -> (x-y=w807:dbl)
                n629 = Greater Or Equal?(x=w807, y=0.0) -> (x >= y?=w812:bool)
                n630 = case shown="假" w812 {
                  tunnel: w807 -> [w820 _]
                  tunnel: w808 -> [w818 _]
                  tunnel: w807 -> [w817 _]
                  frame False {
                    n631 = Greater Or Equal?(x=w817, y=w818) -> (x >= y?=w819:bool)
                    n632 = case shown="真" w819 {
                      tunnel: w820 -> [_ w823]
                      frame False {
                      }
                      frame True {
                        n633 = local read "传感器特性"() -> (w824:cluster{dbl[], dbl[]}[])
                        n634 = local read "初始化"() -> (w822:bool[])
                        n635 = for "For循环" {
                          tunnel: w824 -> [w832] mode=indexing
                          tunnel: [w831] -> w825 mode=indexing
                          tunnel: w823 -> [w830]
                          tunnel: w822 -> [w829] mode=indexing
                          tunnel: [w828] -> w821 mode=indexing
                          i -> [w833]
                          n636 = case shown="9" w833 {
                            tunnel: w832 -> [w835 w846 w860 w876]
                            tunnel: [w835 w844 w858 w872] -> w831
                            tunnel: w830 -> [_ w842 w856 w870]
                            tunnel: w829 -> [w834 w838 w852 w866]
                            tunnel: [w834 FALSE ("布尔") FALSE ("布尔") FALSE ("布尔")] -> w828
                            tunnel: 2 -> [_ w837 w851 w865]
                            tunnel: 2 -> [_ w840 w854 w868]
                            frame Default {
                            }
                            frame 9 {
                              n637 = Unbundle(w846) -> (w849:dbl[], w845:dbl[])
                              n638 = global read "Global.vi" "工位二T1"() -> (w839:dbl)
                              n639 = call-poly <userlib>:"MGI Running Average.vi"("Averaging Size"=w840, "Initialize? (F)"=w838, "Value"=w842) -> ("Average"=w841:dbl)  [unwired: 8 in]
                              n640 = call-poly <userlib>:"MGI Running Average.vi"("Averaging Size"=w837, "Initialize? (F)"=w838, "Value"=w839) -> ("Average"=w836:dbl)  [unwired: 8 in]
                              n641 = Build Array (concatenate)(w845, w836) -> (w847:dbl[])
                              n642 = Build Array (concatenate)(w849, w841) -> (w848:dbl[])
                              n643 = Bundle(w848, w847) -> (w844:cluster{dbl[], dbl[]})  [unwired: 1 in]
                            }
                            frame 10 {
                              n644 = Unbundle(w860) -> (w863:dbl[], w859:dbl[])
                              n645 = global read "Global.vi" "工位二T2"() -> (w853:dbl)
                              n646 = call-poly <userlib>:"MGI Running Average.vi"("Averaging Size"=w854, "Initialize? (F)"=w852, "Value"=w856) -> ("Average"=w855:dbl)  [unwired: 8 in]
                              n647 = call-poly <userlib>:"MGI Running Average.vi"("Averaging Size"=w851, "Initialize? (F)"=w852, "Value"=w853) -> ("Average"=w850:dbl)  [unwired: 8 in]
                              n648 = Build Array (concatenate)(w859, w850) -> (w861:dbl[])
                              n649 = Build Array (concatenate)(w863, w855) -> (w862:dbl[])
                              n650 = Bundle(w862, w861) -> (w858:cluster{dbl[], dbl[]})  [unwired: 1 in]
                            }
                            frame 11 {
                              n651 = Unbundle(w876) -> (w879:dbl[], w875:dbl[])
                              n652 = global read "Global.vi" "工位二T1"() -> (w874:dbl)
                              n653 = global read "Global.vi" "工位二T2"() -> (w873:dbl)
                              n654 = call-poly <userlib>:"MGI Running Average.vi"("Averaging Size"=w868, "Initialize? (F)"=w866, "Value"=w870) -> ("Average"=w869:dbl)  [unwired: 8 in]
                              n655 = Add(x=w874, y=w873) -> (x+y=w867:dbl)
                              n656 = call-poly <userlib>:"MGI Running Average.vi"("Averaging Size"=w865, "Initialize? (F)"=w866, "Value"=w867) -> ("Average"=w864:dbl)  [unwired: 8 in]
                              n657 = Build Array (concatenate)(w875, w864) -> (w877:dbl[])
                              n658 = Build Array (concatenate)(w879, w869) -> (w878:dbl[])
                              n659 = Bundle(w878, w877) -> (w872:cluster{dbl[], dbl[]})  [unwired: 1 in]
                            }
                          }
                        }
                        n660 = local write "初始化"(w821) -> ()
                        n661 = local write "传感器特性"(w825) -> ()
                      }
                    }
                    n662 = call "工位暂停.vi"("枚举"=enum16{"Read", "Write"}."Write", "工位"=enum16{"工位一", "工位二"}."工位二", "Status_Write"=i16 0) -> ()  [unwired: 8 in, 1 out]
                  }
                  frame True {
                    n663 = call "设备状态.vi"("枚举"=enum16{"Read", "Write"}."Write", "工位"=enum16{"工位一", "工位二"}."工位二", "Status_Write"=i16 316) -> ()  [unwired: 8 in, 1 out]
                  }
                }
              }
              frame 316 {
                n664 = global write "Global.vi" "工位占空比采集"(FALSE ("工位二占空比采集")) -> ()
                n665 = local write "STEP"("复检判定" ("STEP")) -> ()
              }
              frame 401 {
                n666 = call "设备状态.vi"("枚举"=enum16{"Read", "Write"}."Write", "工位"=enum16{"工位一", "工位二"}."工位二", "Status_Write"=i16 10) -> ()  [unwired: 8 in, 1 out]
              }
              frame 500 {
                n667 = global read "Global.vi" "动态优化完成"() -> (w888:bool)
                n668 = case shown="真" w888 {
                  frame False {
                    n669 = call "传感器数据.vi"() -> ("传感器读数"=w901:T6)  [unwired: 11 in]
                    n670 = Unbundle By Name(w901) -> ("工位二驱动伺服位移"=w903:sgl)
                    n671 = local read "动优化态前"() -> (w902:cluster{dbl[], dbl[]}[])
                    n672 = local read "初始化 3"() -> (w900:bool[])
                    n673 = for "For循环" {
                      tunnel: [w910] -> w898 mode=indexing
                      tunnel: w903 -> [w909]
                      tunnel: w902 -> [w908] mode=indexing
                      tunnel: w900 -> [w906] mode=indexing
                      tunnel: [w905] -> w899 mode=indexing
                      i -> [w907]
                      n674 = case shown="0" w907 {
                        tunnel: [w912 w920 w930 w942 w954] -> w910
                        tunnel: w909 -> [_ w915 w925 w933 w945]
                        tunnel: w908 -> [w912 w918 w927 w939 w951]
                        tunnel: w906 -> [w911 w914 w924 w936 w948]
                        tunnel: [w911 FALSE ("布尔") FALSE ("布尔") FALSE ("布尔") FALSE ("布尔")] -> w905
                        tunnel: 10 ("rank") -> [_ _ _ w935 w947]
                        frame Default {
                        }
                        frame 0 {
                          n675 = global read "Global.vi" "工位二T1"() -> (w913:dbl)
                          n676 = call <vilib>:"Median Filter PtByPt.vi"("initialize"=w914) -> ()  [unwired: 3 in, 2 out]
                          n677 = Unbundle(w918) -> (w917:dbl[], w919:dbl[])
                          n678 = call <vilib>:"Median Filter PtByPt.vi"("initialize"=w914, "x"=w913) -> ()  [unwired: 2 in, 2 out]
                          n679 = Build Array (concatenate)(w917, w915) -> (w922:dbl[])
                          n680 = Build Array (concatenate)(w919, w913) -> (w921:dbl[])
                          n681 = Bundle(w922, w921) -> (w920:cluster{dbl[], dbl[]})  [unwired: 1 in]
                        }
                        frame 1 {
                          n682 = call <vilib>:"Median Filter PtByPt.vi"("initialize"=w924) -> ()  [unwired: 3 in, 2 out]
                          n683 = Unbundle(w927) -> (w929:dbl[], w928:dbl[])
                          n684 = global read "Global.vi" "工位二T2"() -> (w923:dbl)
                          n685 = Build Array (concatenate)(w929, w925) -> (w932:dbl[])
                          n686 = call <vilib>:"Median Filter PtByPt.vi"("initialize"=w924, "x"=w923) -> ()  [unwired: 2 in, 2 out]
                          n687 = Build Array (concatenate)(w928, w923) -> (w931:dbl[])
                          n688 = Bundle(w932, w931) -> (w930:cluster{dbl[], dbl[]})  [unwired: 1 in]
                        }
                        frame 2 {
                          n689 = global read "Global.vi" "工位二P"() -> (w937:dbl)
                          n690 = Unbundle(w939) -> (w941:dbl[], w940:dbl[])
                          n691 = call <vilib>:"Median Filter PtByPt.vi"("initialize"=w936, "rank"=w935, "x"=w937) -> ("Filtered x"=w934:dbl)  [unwired: 1 in, 1 out]
                          n692 = call-poly <userlib>:"MGI Running Average.vi"("Averaging Size"=w935, "Initialize? (F)"=w936, "Value"=w937) -> ()  [unwired: 8 in, 1 out]
                          n693 = Build Array (concatenate)(w940, w934) -> (w943:dbl[])
                          n694 = Build Array (concatenate)(w941, w933) -> (w944:dbl[])
                          n695 = Bundle(w944, w943) -> (w942:cluster{dbl[], dbl[]})  [unwired: 1 in]
                        }
                        frame 3 {
                          n696 = global read "Global.vi" "工位二S"() -> (w949:dbl)
                          n697 = Unbundle(w951) -> (w953:dbl[], w952:dbl[])
                          n698 = call <vilib>:"Median Filter PtByPt.vi"("initialize"=w948, "rank"=w947, "x"=w949) -> ("Filtered x"=w946:dbl)  [unwired: 1 in, 1 out]
                          n699 = call-poly <userlib>:"MGI Running Average.vi"("Averaging Size"=w947, "Initialize? (F)"=w948, "Value"=w949) -> ()  [unwired: 8 in, 1 out]
                          n700 = Build Array (concatenate)(w953, w945) -> (w956:dbl[])
                          n701 = Build Array (concatenate)(w952, w946) -> (w955:dbl[])
                          n702 = Bundle(w956, w955) -> (w954:cluster{dbl[], dbl[]})  [unwired: 1 in]
                        }
                      }
                    }
                    n703 = local write "初始化 3"(w899) -> ()
                    n704 = local write "动优化态前"(w898) -> ()
                    n705 = call "VRES值.vi"("XY"=w898, "索引1"=2, "索引2"=3) -> ("XY图 2"=w897:cluster{dbl[], dbl[]}[])  [unwired: 16 in]
                    n706 = Index Array(array=w897, index=8 ("索引")) -> (element=→"VRES_cW":cluster{dbl[], dbl[]})
                  }
                  frame True {
                    n707 = call "传感器数据.vi"() -> ("传感器读数"=w960:T6)  [unwired: 11 in]
                    n708 = Unbundle By Name(w960) -> ("工位二驱动伺服位移"=w962:sgl)
                    n709 = local read "可信度检测"() -> (w961:cluster{dbl[], dbl[]}[])
                    n710 = local read "初始化 2"() -> (w959:bool[])
                    n711 = for "For循环" {
                      tunnel: [w969] -> w957 mode=indexing
                      tunnel: w962 -> [w968]
                      tunnel: w961 -> [w967] mode=indexing
                      tunnel: w959 -> [w965] mode=indexing
                      tunnel: [w964] -> w958 mode=indexing
                      i -> [w966]
                      n712 = case shown="2" w966 {
                        tunnel: [w971 w979 w989 w1003] -> w969
                        tunnel: w968 -> [_ w974 w984 w992]
                        tunnel: w967 -> [w971 w977 w986 w1000]
                        tunnel: w965 -> [w970 w973 w983 w994]
                        tunnel: [w970 FALSE ("布尔") FALSE ("布尔") FALSE ("布尔")] -> w964
                        tunnel: 10 ("rank") -> [_ _ _ w995]
                        frame Default {
                        }
                        frame 0 {
                          n713 = global read "Global.vi" "工位二T1"() -> (w972:dbl)
                          n714 = call <vilib>:"Median Filter PtByPt.vi"("initialize"=w973) -> ()  [unwired: 3 in, 2 out]
                          n715 = Unbundle(w977) -> (w976:dbl[], w978:dbl[])
                          n716 = Build Array (concatenate)(w976, w974) -> (w981:dbl[])
                          n717 = call <vilib>:"Median Filter PtByPt.vi"("x"=w972) -> ()  [unwired: 3 in, 2 out]
                          n718 = Build Array (concatenate)(w978, w972) -> (w980:dbl[])
                          n719 = Bundle(w981, w980) -> (w979:cluster{dbl[], dbl[]})  [unwired: 1 in]
                        }
                        frame 1 {
                          n720 = global read "Global.vi" "工位二T2"() -> (w982:dbl)
                          n721 = Unbundle(w986) -> (w988:dbl[], w987:dbl[])
                          n722 = Build Array (concatenate)(w988, w984) -> (w991:dbl[])
                          n723 = call <vilib>:"Median Filter PtByPt.vi"("initialize"=w983, "x"=w982) -> ()  [unwired: 2 in, 2 out]
                          n724 = Build Array (concatenate)(w987, w982) -> (w990:dbl[])
                          n725 = Bundle(w991, w990) -> (w989:cluster{dbl[], dbl[]})  [unwired: 1 in]
                        }
                        frame 2 {
                          n726 = global read "Global.vi" "工位二P"() -> (w997:dbl)
                          n727 = global read "Global.vi" "工位二S"() -> (w998:dbl)
                          n728 = Unbundle(w1000) -> (w1002:dbl[], w1001:dbl[])
                          n729 = Build Array (concatenate)(w1002, w992) -> (w1005:dbl[])
                          n730 = call "Calc_Vres.vi"("S_Data in"=w998, "P_Data in"=w997) -> ("Vres"=w996:dbl)  [unwired: 7 in, 2 out]
                          n731 = call <vilib>:"Median Filter PtByPt.vi"("initialize"=w994, "rank"=w995, "x"=w996) -> ("Filtered x"=w993:dbl)  [unwired: 1 in, 1 out]
                          n732 = Build Array (concatenate)(w1001, w993) -> (w1004:dbl[])
                          n733 = call-poly <userlib>:"MGI Running Average.vi"("Averaging Size"=w995, "Initialize? (F)"=w994, "Value"=w996) -> ()  [unwired: 8 in, 1 out]
                          n734 = Bundle(w1005, w1004) -> (w1003:cluster{dbl[], dbl[]})  [unwired: 1 in]
                        }
                      }
                    }
                    n735 = local write "初始化 2"(w958) -> ()
                    n736 = local write "可信度检测"(w957) -> ()
                  }
                }
                n737 = call "浮动通知.vi"("通知内容"="可信度检测" ("Status")) -> ()  [unwired: 11 in]
                n738 = local read "initialize 2"() -> (w891:bool)
                n739 = case shown="0" 0 {
                  tunnel: [w1006 FALSE ("initialize 2")] -> w890
                  tunnel: w891 -> [w1006 _]
                  frame Default {
                  }
                  frame 0 {
                  }
                }
                n740 = local write "initialize 2"(w890) -> ()
              }
              frame 501 {
                n741 = global read "Global.vi" "动态优化完成"() -> (w1008:bool)
                n742 = case shown="真" w1008 {
                  frame False {
                    n743 = call "传感器数据.vi"() -> ("传感器读数"=w1021:T6)  [unwired: 11 in]
                    n744 = Unbundle By Name(w1021) -> ("工位二驱动伺服位移"=w1016:sgl)
                    n745 = local read "动优化态前"() -> (w1022:cluster{dbl[], dbl[]}[])
                    n746 = local read "初始化 3"() -> (w1020:bool[])
                    n747 = for "For循环" {
                      tunnel: [w1029] -> w1017 mode=indexing
                      tunnel: w1016 -> [w1028]
                      tunnel: w1022 -> [w1027] mode=indexing
                      tunnel: w1020 -> [w1025] mode=indexing
                      tunnel: [w1024] -> w1019 mode=indexing
                      i -> [w1026]
                      n748 = case shown="7" w1026 {
                        tunnel: [w1031 w1039 w1049 w1061 w1073] -> w1029
                        tunnel: w1028 -> [_ w1034 w1044 w1056 w1064]
                        tunnel: w1027 -> [w1031 w1036 w1046 w1058 w1070]
                        tunnel: w1025 -> [w1030 w1033 w1043 w1054 w1067]
                        tunnel: [w1030 FALSE ("布尔") FALSE ("布尔") FALSE ("布尔") FALSE ("布尔")] -> w1024
                        tunnel: 10 ("rank") -> [_ _ _ w1052 w1066]
                        frame Default {
                        }
                        frame 4 {
                          n749 = global read "Global.vi" "工位二T1"() -> (w1032:dbl)
                          n750 = call <vilib>:"Median Filter PtByPt.vi"("initialize"=w1033) -> ()  [unwired: 3 in, 2 out]
                          n751 = Unbundle(w1036) -> (w1038:dbl[], w1037:dbl[])
                          n752 = Build Array (concatenate)(w1038, w1034) -> (w1041:dbl[])
                          n753 = call <vilib>:"Median Filter PtByPt.vi"("initialize"=w1033, "x"=w1032) -> ()  [unwired: 2 in, 2 out]
                          n754 = Build Array (concatenate)(w1037, w1032) -> (w1040:dbl[])
                          n755 = Bundle(w1041, w1040) -> (w1039:cluster{dbl[], dbl[]})  [unwired: 1 in]
                        }
                        frame 5 {
                          n756 = global read "Global.vi" "工位二T2"() -> (w1042:dbl)
                          n757 = Unbundle(w1046) -> (w1048:dbl[], w1047:dbl[])
                          n758 = call <vilib>:"Median Filter PtByPt.vi"("initialize"=w1043) -> ()  [unwired: 3 in, 2 out]
                          n759 = Build Array (concatenate)(w1048, w1044) -> (w1051:dbl[])
                          n760 = call <vilib>:"Median Filter PtByPt.vi"("initialize"=w1043, "x"=w1042) -> ()  [unwired: 2 in, 2 out]
                          n761 = Build Array (concatenate)(w1047, w1042) -> (w1050:dbl[])
                          n762 = Bundle(w1051, w1050) -> (w1049:cluster{dbl[], dbl[]})  [unwired: 1 in]
                        }
                        frame 6 {
                          n763 = call <vilib>:"Median Filter PtByPt.vi"("initialize"=w1054, "rank"=w1052, "x"=w1056) -> ()  [unwired: 1 in, 2 out]
                          n764 = Unbundle(w1058) -> (w1060:dbl[], w1059:dbl[])
                          n765 = global read "Global.vi" "工位二P"() -> (w1055:dbl)
                          n766 = Build Array (concatenate)(w1060, w1056) -> (w1063:dbl[])
                          n767 = call <vilib>:"Median Filter PtByPt.vi"("initialize"=w1054, "rank"=w1052, "x"=w1055) -> ()  [unwired: 1 in, 2 out]
                          n768 = call-poly <userlib>:"MGI Running Average.vi"("Averaging Size"=w1052, "Initialize? (F)"=w1054, "Value"=w1055) -> ("Average"=w1053:dbl)  [unwired: 8 in]
                          n769 = Build Array (concatenate)(w1059, w1053) -> (w1062:dbl[])
                          n770 = Bundle(w1063, w1062) -> (w1061:cluster{dbl[], dbl[]})  [unwired: 1 in]
                        }
                        frame 7 {
                          n771 = global read "Global.vi" "工位二S"() -> (w1068:dbl)
                          n772 = Unbundle(w1070) -> (w1072:dbl[], w1071:dbl[])
                          n773 = call <vilib>:"Median Filter PtByPt.vi"("initialize"=w1067, "rank"=w1066, "x"=w1068) -> ("Filtered x"=w1065:dbl)  [unwired: 1 in, 1 out]
                          n774 = call-poly <userlib>:"MGI Running Average.vi"("Averaging Size"=w1066, "Initialize? (F)"=w1067, "Value"=w1068) -> ()  [unwired: 8 in, 1 out]
                          n775 = Build Array (concatenate)(w1071, w1065) -> (w1074:dbl[])
                          n776 = Build Array (concatenate)(w1072, w1064) -> (w1075:dbl[])
                          n777 = Bundle(w1075, w1074) -> (w1073:cluster{dbl[], dbl[]})  [unwired: 1 in]
                        }
                      }
                    }
                    n778 = local write "初始化 3"(w1019) -> ()
                    n779 = local write "动优化态前"(w1017) -> ()
                    n780 = call "VRES值.vi"("XY"=w1017, "索引1"=6, "索引2"=7) -> ("XY图 2"=w1018:cluster{dbl[], dbl[]}[])  [unwired: 16 in]
                    n781 = Index Array(array=w1018, index=8 ("索引")) -> (element=→"vRES_cCW":cluster{dbl[], dbl[]})
                  }
                  frame True {
                    n782 = call "传感器数据.vi"() -> ("传感器读数"=w1080:T6)  [unwired: 11 in]
                    n783 = Unbundle By Name(w1080) -> ("工位二驱动伺服位移"=w1076:sgl)
                    n784 = local read "可信度检测"() -> (w1081:cluster{dbl[], dbl[]}[])
                    n785 = local read "初始化 2"() -> (w1079:bool[])
                    n786 = for "For循环" {
                      tunnel: [w1088] -> w1077 mode=indexing
                      tunnel: w1076 -> [w1087]
                      tunnel: w1081 -> [w1086] mode=indexing
                      tunnel: w1079 -> [w1084] mode=indexing
                      tunnel: [w1083] -> w1078 mode=indexing
                      i -> [w1085]
                      n787 = case shown="4" w1085 {
                        tunnel: [w1090 w1098 w1108 w1122] -> w1088
                        tunnel: w1087 -> [_ w1093 w1103 w1112]
                        tunnel: w1086 -> [w1090 w1095 w1105 w1119]
                        tunnel: w1084 -> [w1089 w1092 w1102 w1114]
                        tunnel: [w1089 FALSE ("布尔") FALSE ("布尔") FALSE ("布尔")] -> w1083
                        tunnel: 10 ("rank") -> [_ _ _ w1111]
                        frame Default {
                        }
                        frame 3 {
                          n788 = call <vilib>:"Median Filter PtByPt.vi"("initialize"=w1092) -> ()  [unwired: 3 in, 2 out]
                          n789 = Unbundle(w1095) -> (w1097:dbl[], w1096:dbl[])
                          n790 = global read "Global.vi" "工位二T1"() -> (w1091:dbl)
                          n791 = Build Array (concatenate)(w1097, w1093) -> (w1100:dbl[])
                          n792 = call <vilib>:"Median Filter PtByPt.vi"("initialize"=w1092, "x"=w1091) -> ()  [unwired: 2 in, 2 out]
                          n793 = Build Array (concatenate)(w1096, w1091) -> (w1099:dbl[])
                          n794 = Bundle(w1100, w1099) -> (w1098:cluster{dbl[], dbl[]})  [unwired: 1 in]
                        }
                        frame 4 {
                          n795 = global read "Global.vi" "工位二T2"() -> (w1101:dbl)
                          n796 = call <vilib>:"Median Filter PtByPt.vi"("initialize"=w1102) -> ()  [unwired: 3 in, 2 out]
                          n797 = Unbundle(w1105) -> (w1107:dbl[], w1106:dbl[])
                          n798 = Build Array (concatenate)(w1107, w1103) -> (w1110:dbl[])
                          n799 = call <vilib>:"Median Filter PtByPt.vi"("initialize"=w1102, "x"=w1101) -> ()  [unwired: 2 in, 2 out]
                          n800 = Build Array (concatenate)(w1106, w1101) -> (w1109:dbl[])
                          n801 = Bundle(w1110, w1109) -> (w1108:cluster{dbl[], dbl[]})  [unwired: 1 in]
                        }
                        frame 5 {
                          n802 = global read "Global.vi" "工位二P"() -> (w1116:dbl)
                          n803 = global read "Global.vi" "工位二S"() -> (w1117:dbl)
                          n804 = call <vilib>:"Median Filter PtByPt.vi"("initialize"=w1114, "rank"=w1111, "x"=w1112) -> ()  [unwired: 1 in, 2 out]
                          n805 = Unbundle(w1119) -> (w1121:dbl[], w1120:dbl[])
                          n806 = Build Array (concatenate)(w1121, w1112) -> (w1124:dbl[])
                          n807 = call "Calc_Vres.vi"("S_Data in"=w1117, "P_Data in"=w1116) -> ("Vres"=w1115:dbl)  [unwired: 7 in, 2 out]
                          n808 = call <vilib>:"Median Filter PtByPt.vi"("initialize"=w1114, "rank"=w1111, "x"=w1115) -> ()  [unwired: 1 in, 2 out]
                          n809 = call-poly <userlib>:"MGI Running Average.vi"("Averaging Size"=w1111, "Initialize? (F)"=w1114, "Value"=w1115) -> ("Average"=w1113:dbl)  [unwired: 8 in]
                          n810 = Build Array (concatenate)(w1120, w1113) -> (w1123:dbl[])
                          n811 = Bundle(w1124, w1123) -> (w1122:cluster{dbl[], dbl[]})  [unwired: 1 in]
                        }
                      }
                    }
                    n812 = local write "可信度检测"(w1077) -> ()
                    n813 = local write "初始化 2"(w1078) -> ()
                  }
                }
                n814 = local read "initialize"() -> (w1011:bool)
                n815 = for "For循环" {
                  N: 5 -> [_]
                  tunnel: w1011 -> [w1126]
                  tunnel: [w1127] -> w1010
                  i -> [w1125]
                  n816 = case shown="0" w1125 {
                    tunnel: [w1128 FALSE ("initialize")] -> w1127
                    tunnel: w1126 -> [w1128 _]
                    frame Default {
                    }
                    frame 0 {
                    }
                  }
                }
                n817 = local write "initialize"(w1010) -> ()
              }
              frame 502 {
                n818 = global read "Global.vi" "动态优化完成"() -> (w1130:bool)
                n819 = case shown="假" w1130 {
                  frame False {
                    n820 = stacked-sequence {
                      frame #0 {
                        n821 = local read "动优化态前"() -> (w1131:cluster{dbl[], dbl[]}[])
                        n822 = for "For循环" {
                          tunnel: w1131 -> [w1132] mode=indexing
                          i -> [w1133]
                          n823 = Unbundle(w1132) -> (w1134:dbl[])  [unwired: 1 out]
                          n824 = case shown="1" w1133 {
                            tunnel: w1134 -> [_ w1135 w1136 w1137 w1138 w1139 w1140 w1141 w1142]
                            frame Default {
                            }
                            frame 0 {
                              n825 = local write "T1_CW"(w1135) -> ()
                            }
                            frame 1 {
                              n826 = local write "T2_CW"(w1136) -> ()
                            }
                            frame 2 {
                              n827 = local write "P_CW"(w1137) -> ()
                            }
                            frame 3 {
                              n828 = local write "S_CW"(w1138) -> ()
                            }
                            frame 4 {
                              n829 = local write "T1_CCw"(w1139) -> ()
                            }
                            frame 5 {
                              n830 = local write "T2_CCw"(w1140) -> ()
                            }
                            frame 6 {
                              n831 = local write "P_CCw"(w1141) -> ()
                            }
                            frame 7 {
                              n832 = local write "S_CCw"(w1142) -> ()
                            }
                          }
                        }
                      }
                      frame #1 {
                        n833 = local read "T1_CCw"() -> (w1147:dbl[])
                        n834 = local read "T2_CCw"() -> (w1149:dbl[])
                        n835 = local read "T1_CW"() -> (w1145:dbl[])
                        n836 = local read "T2_CW"() -> (w1148:dbl[])
                        n837 = Build Array(w1148, w1149) -> (w1150:dbl[][])
                        n838 = local read "SENSOR"() -> (w1151:T1)
                        n839 = call-poly <userlib>:"MGI Average.vi"("Double[][]"=w1150, "Ignore NaN? (F)"=TRUE) -> ("Average"=w1153:dbl)
                        n840 = Build Array(w1145, w1147) -> (w1146:dbl[][])
                        n841 = local read "P_CCw"() -> (w1154:dbl[])
                        n842 = local read "S_CCw"() -> (w1156:dbl[])
                        n843 = local read "S_CW"() -> (w1157:dbl[])
                        n844 = local read "P_CW"() -> (w1155:dbl[])
                        n845 = call-poly <userlib>:"MGI Average.vi"("Double[][]"=w1146, "Ignore NaN? (F)"=TRUE) -> ("Average"=w1152:dbl)
                        n846 = call "动态优化.vi"("S_CCw"=w1156, "S_Cw"=w1157, "P_CCw"=w1154, "SENSOR"=w1151, "P_Cw"=w1155, "T2_AV(%)"=w1153, "T1_AV(%)"=w1152) -> ("OK？"=w1158:bool)  [unwired: 4 in]
                        n847 = case shown="真" w1158 {
                          selector: w1158 -> [_ w1166]
                          frame False {
                          }
                          frame True {
                            n848 = global read "Global.vi" "8点复测"() -> (w1162:bool)
                            n849 = global read "Global.vi" "动态优化复测"() -> (w1165:bool)
                            n850 = global write "Global.vi" "动态优化完成"(w1166) -> ()
                            n851 = Select(t="动态优化", s=w1165, f="复测") -> (s? t:f=w1161:string)
                            n852 = Select(t=w1161, s=w1162, f="复测判定") -> (s? t:f=w1159:string)
                            n853 = local write "STEP"(w1159) -> ()
                          }
                        }
                      }
                    }
                  }
                  frame True {
                    w1171 = FALSE ("工位二占空比采集")
                    n854 = local read "可信度检测"() -> (w1172:cluster{dbl[], dbl[]}[])
                    n855 = for "For循环" {
                      tunnel: w1172 -> [w1173] mode=indexing
                      i -> [w1174]
                      n856 = Unbundle(w1173) -> (w1175:dbl[])  [unwired: 1 out]
                      n857 = case shown="5" w1174 {
                        tunnel: w1175 -> [_ w1176 w1177 _ w1179 w1180 _]
                        tunnel: w1173 -> [_ _ _ w1178 _ _ w1181]
                        frame Default {
                        }
                        frame 0 {
                          n858 = local write "T1_CW"(w1176) -> ()
                        }
                        frame 1 {
                          n859 = local write "T2_CW"(w1177) -> ()
                        }
                        frame 2 {
                          n860 = local write "VRES_cW"(w1178) -> ()
                        }
                        frame 3 {
                          n861 = local write "T1_CCw"(w1179) -> ()
                        }
                        frame 4 {
                          n862 = local write "T2_CCw"(w1180) -> ()
                        }
                        frame 5 {
                          n863 = local write "vRES_cCW"(w1181) -> ()
                        }
                      }
                    }
                    n864 = global write "Global.vi" "P/S采集"(w1171) -> ()
                    n865 = global write "Global.vi" "工位占空比采集"(w1171) -> ()
                    n866 = global read "Global.vi" "8点复测"() -> (w1170:bool)
                    n867 = Select(t="复测", s=w1170, f="复测判定") -> (s? t:f=w1168:string)
                    n868 = local write "STEP"(w1168) -> ()
                  }
                }
              }
              frame 505 {
                w1182 = TRUE ("initialize")
                n869 = local write "initialize"(w1182) -> ()
                n870 = local write "initialize 2"(w1182) -> ()
              }
              frame 511 {
                n871 = stacked-sequence {
                  frame #0 {
                    n872 = Wait (ms)(milliseconds to wait=u32 500 ("等待时间（毫秒）")) -> ()  [unwired: 1 out]
                  }
                  frame #1 {
                    w1193 = 10171 items=["上升"=10280, "下降"=10171] ("starting edge2")
                    w1192 = 10280 items=["上升"=10280, "下降"=10171] ("starting edge1")
                    w1194 = 10171 items=["上升"=10280, "下降"=10171] ("starting edge2")
                    w1195 = 10280 items=["上升"=10280, "下降"=10171] ("starting edge1")
                    w1202 = 10171 items=["上升"=10280, "下降"=10171] ("starting edge")
                    w1204 = 10171 items=["上升"=10280, "下降"=10171] ("starting edge")
                    w1203 = 10280 items=["上升"=10280, "下降"=10171] ("starting edge")
                    w1205 = 10280 items=["上升"=10280, "下降"=10171] ("starting edge")
                    n873 = local read "VRES_cW"() -> (w1201:cluster{dbl[], dbl[]})
                    n874 = Unbundle(w1201) -> (w1199:dbl[], w1198:dbl[])
                    n875 = call "占空比测量.vi"("计数器"=tag "Dev2/ctr2", "starting edge1"=w1205, "starting edge2"=w1204) -> ("占空比2(%)"=w1208:dbl)  [unwired: 4 in, 3 out]
                    n876 = call "占空比测量.vi"("计数器"=tag "Dev2/ctr3", "starting edge1"=w1203, "starting edge2"=w1202) -> ("占空比(%)"=w1207:dbl)  [unwired: 4 in, 3 out]
                    n877 = Threshold 1D Array(2:90.0 ("分数索引或x"), 3:w1199) -> (0:w1197:dbl)  [unwired: 1 in]
                    n878 = call "占空比测量.vi"("计数器"=tag "Dev2/ctr1", "starting edge1"=w1195, "starting edge2"=w1194) -> ("占空比2(%)"=w1190:dbl)  [unwired: 4 in, 3 out]
                    n879 = call "占空比测量.vi"("计数器"=tag "Dev2/ctr0", "starting edge1"=w1192, "starting edge2"=w1193) -> ("占空比2(%)"=w1189:dbl)  [unwired: 4 in, 3 out]
                    n880 = call "Calc_Vres.vi"("S_Data in"=w1207, "P_Data in"=w1208) -> ("Vres"=w1187:dbl)  [unwired: 7 in, 2 out]
                    n881 = Interpolate 1D Array(1:w1197, 2:w1198) -> (0:w1185:dbl)
                    n882 = Subtract(x=w1190, y=w1189) -> (x-y=→"T1-T2_90°":dbl)
                    n883 = Max & Min(x=w1185, y=w1187) -> (max(x,y)=w1186:dbl)  [unwired: 1 out]
                    n884 = local write "Vres_90°"(w1186) -> ()
                  }
                  frame #2 {
                    n885 = call "设备状态.vi"("枚举"=enum16{"Read", "Write"}."Write", "工位"=enum16{"工位一", "工位二"}."工位二", "Status_Write"=i16 512) -> ()  [unwired: 8 in, 1 out]
                  }
                }
                n886 = call "浮动通知.vi"("通知内容"="正向复测！" ("Status")) -> ()  [unwired: 11 in]
              }
              frame 513 {
                n887 = stacked-sequence {
                  frame #0 {
                    n888 = Wait (ms)(milliseconds to wait=u32 500 ("等待时间（毫秒）")) -> ()  [unwired: 1 out]
                  }
                  frame #1 {
                    w1222 = 10171 items=["上升"=10280, "下降"=10171] ("starting edge2")
                    w1221 = 10280 items=["上升"=10280, "下降"=10171] ("starting edge1")
                    w1223 = 10171 items=["上升"=10280, "下降"=10171] ("starting edge2")
                    w1224 = 10280 items=["上升"=10280, "下降"=10171] ("starting edge1")
                    w1231 = 10171 items=["上升"=10280, "下降"=10171] ("starting edge")
                    w1232 = 10280 items=["上升"=10280, "下降"=10171] ("starting edge")
                    w1233 = 10171 items=["上升"=10280, "下降"=10171] ("starting edge")
                    w1234 = 10280 items=["上升"=10280, "下降"=10171] ("starting edge")
                    n889 = local read "VRES_cW"() -> (w1230:cluster{dbl[], dbl[]})
                    n890 = Unbundle(w1230) -> (w1228:dbl[], w1227:dbl[])
                    n891 = call "占空比测量.vi"("计数器"=tag "Dev2/ctr6", "starting edge1"=w1234, "starting edge2"=w1233) -> ("占空比2(%)"=w1236:dbl)  [unwired: 4 in, 3 out]
                    n892 = call "占空比测量.vi"("计数器"=tag "Dev2/ctr7", "starting edge1"=w1232, "starting edge2"=w1231) -> ("占空比(%)"=w1235:dbl)  [unwired: 4 in, 3 out]
                    n893 = Threshold 1D Array(2:180.0 ("分数索引或x"), 3:w1228) -> (0:w1226:dbl)  [unwired: 1 in]
                    n894 = call "Calc_Vres.vi"("S_Data in"=w1235, "P_Data in"=w1236) -> ("Vres"=w1215:dbl)  [unwired: 7 in, 2 out]
                    n895 = Interpolate 1D Array(1:w1226, 2:w1227) -> (0:w1214:dbl)
                    n896 = call "占空比测量.vi"("计数器"=tag "Dev2/ctr1", "starting edge1"=w1224, "starting edge2"=w1223) -> ("占空比2(%)"=w1219:dbl)  [unwired: 4 in, 3 out]
                    n897 = call "占空比测量.vi"("计数器"=tag "Dev2/ctr0", "starting edge1"=w1221, "starting edge2"=w1222) -> ("占空比2(%)"=w1218:dbl)  [unwired: 4 in, 3 out]
                    n898 = Subtract(x=w1219, y=w1218) -> (x-y=→"T1-T2_180°":dbl)
                    n899 = Max & Min(x=w1214, y=w1215) -> (max(x,y)=w1216:dbl)  [unwired: 1 out]
                    n900 = local write "Vres_180°"(w1216) -> ()
                  }
                  frame #2 {
                    n901 = call "设备状态.vi"("枚举"=enum16{"Read", "Write"}."Write", "工位"=enum16{"工位一", "工位二"}."工位二", "Status_Write"=i16 514) -> ()  [unwired: 8 in, 1 out]
                  }
                }
              }
              frame 515 {
                n902 = stacked-sequence {
                  frame #0 {
                    n903 = Wait (ms)(milliseconds to wait=u32 500 ("等待时间（毫秒）")) -> ()  [unwired: 1 out]
                  }
                  frame #1 {
                    w1251 = 10171 items=["上升"=10280, "下降"=10171] ("starting edge2")
                    w1250 = 10280 items=["上升"=10280, "下降"=10171] ("starting edge1")
                    w1252 = 10171 items=["上升"=10280, "下降"=10171] ("starting edge2")
                    w1253 = 10280 items=["上升"=10280, "下降"=10171] ("starting edge1")
                    w1260 = 10171 items=["上升"=10280, "下降"=10171] ("starting edge")
                    w1261 = 10280 items=["上升"=10280, "下降"=10171] ("starting edge")
                    w1262 = 10171 items=["上升"=10280, "下降"=10171] ("starting edge")
                    w1263 = 10280 items=["上升"=10280, "下降"=10171] ("starting edge")
                    n904 = local read "VRES_cW"() -> (w1259:cluster{dbl[], dbl[]})
                    n905 = Unbundle(w1259) -> (w1257:dbl[], w1256:dbl[])
                    n906 = call "占空比测量.vi"("计数器"=tag "Dev2/ctr6", "starting edge1"=w1263, "starting edge2"=w1262) -> ("占空比2(%)"=w1265:dbl)  [unwired: 4 in, 3 out]
                    n907 = call "占空比测量.vi"("计数器"=tag "Dev2/ctr7", "starting edge1"=w1261, "starting edge2"=w1260) -> ("占空比(%)"=w1264:dbl)  [unwired: 4 in, 3 out]
                    n908 = Threshold 1D Array(2:270.0 ("分数索引或x"), 3:w1257) -> (0:w1255:dbl)  [unwired: 1 in]
                    n909 = call "Calc_Vres.vi"("S_Data in"=w1264, "P_Data in"=w1265) -> ("Vres"=w1243:dbl)  [unwired: 7 in, 2 out]
                    n910 = call "占空比测量.vi"("计数器"=tag "Dev2/ctr1", "starting edge1"=w1253, "starting edge2"=w1252) -> ("占空比2(%)"=w1248:dbl)  [unwired: 4 in, 3 out]
                    n911 = call "占空比测量.vi"("计数器"=tag "Dev2/ctr0", "starting edge1"=w1250, "starting edge2"=w1251) -> ("占空比2(%)"=w1247:dbl)  [unwired: 4 in, 3 out]
                    n912 = Interpolate 1D Array(1:w1255, 2:w1256) -> (0:w1244:dbl)
                    n913 = Subtract(x=w1248, y=w1247) -> (x-y=→"T1-T2_270°":dbl)
                    n914 = Max & Min(x=w1244, y=w1243) -> (max(x,y)=w1245:dbl)  [unwired: 1 out]
                    n915 = local write "Vres_270°"(w1245) -> ()
                  }
                  frame #2 {
                    n916 = call "设备状态.vi"("枚举"=enum16{"Read", "Write"}."Write", "工位"=enum16{"工位一", "工位二"}."工位二", "Status_Write"=i16 516) -> ()  [unwired: 8 in, 1 out]
                  }
                }
              }
              frame 517 {
                n917 = stacked-sequence {
                  frame #0 {
                    n918 = Wait (ms)(milliseconds to wait=u32 500 ("等待时间（毫秒）")) -> ()  [unwired: 1 out]
                  }
                  frame #1 {
                    w1280 = 10171 items=["上升"=10280, "下降"=10171] ("starting edge2")
                    w1279 = 10280 items=["上升"=10280, "下降"=10171] ("starting edge1")
                    w1281 = 10171 items=["上升"=10280, "下降"=10171] ("starting edge2")
                    w1282 = 10280 items=["上升"=10280, "下降"=10171] ("starting edge1")
                    w1289 = 10171 items=["上升"=10280, "下降"=10171] ("starting edge")
                    w1290 = 10280 items=["上升"=10280, "下降"=10171] ("starting edge")
                    w1291 = 10171 items=["上升"=10280, "下降"=10171] ("starting edge")
                    w1292 = 10280 items=["上升"=10280, "下降"=10171] ("starting edge")
                    n919 = local read "VRES_cW"() -> (w1288:cluster{dbl[], dbl[]})
                    n920 = Unbundle(w1288) -> (w1286:dbl[], w1285:dbl[])
                    n921 = call "占空比测量.vi"("计数器"=tag "Dev2/ctr6", "starting edge1"=w1292, "starting edge2"=w1291) -> ("占空比2(%)"=w1294:dbl)  [unwired: 4 in, 3 out]
                    n922 = call "占空比测量.vi"("计数器"=tag "Dev2/ctr7", "starting edge1"=w1290, "starting edge2"=w1289) -> ("占空比(%)"=w1293:dbl)  [unwired: 4 in, 3 out]
                    n923 = Threshold 1D Array(2:360.0 ("分数索引或x"), 3:w1286) -> (0:w1284:dbl)  [unwired: 1 in]
                    n924 = call "Calc_Vres.vi"("S_Data in"=w1293, "P_Data in"=w1294) -> ("Vres"=w1272:dbl)  [unwired: 7 in, 2 out]
                    n925 = call "占空比测量.vi"("计数器"=tag "Dev2/ctr4", "starting edge1"=w1282, "starting edge2"=w1281) -> ("占空比2(%)"=w1277:dbl)  [unwired: 4 in, 3 out]
                    n926 = call "占空比测量.vi"("计数器"=tag "Dev2/ctr5", "starting edge1"=w1279, "starting edge2"=w1280) -> ("占空比2(%)"=w1276:dbl)  [unwired: 4 in, 3 out]
                    n927 = Interpolate 1D Array(1:w1284, 2:w1285) -> (0:w1273:dbl)
                    n928 = Subtract(x=w1277, y=w1276) -> (x-y=→"T1-T2_360°":dbl)
                    n929 = Max & Min(x=w1273, y=w1272) -> (max(x,y)=w1274:dbl)  [unwired: 1 out]
                    n930 = local write "Vres_360°"(w1274) -> ()
                  }
                  frame #2 {
                    n931 = call "设备状态.vi"("枚举"=enum16{"Read", "Write"}."Write", "工位"=enum16{"工位一", "工位二"}."工位二", "Status_Write"=i16 520) -> ()  [unwired: 8 in, 1 out]
                  }
                }
              }
              frame 521 {
                n932 = stacked-sequence {
                  frame #0 {
                    n933 = Wait (ms)(milliseconds to wait=u32 500 ("等待时间（毫秒）")) -> ()  [unwired: 1 out]
                  }
                  frame #1 {
                    w1310 = 10171 items=["上升"=10280, "下降"=10171] ("starting edge2")
                    w1309 = 10280 items=["上升"=10280, "下降"=10171] ("starting edge1")
                    w1311 = 10171 items=["上升"=10280, "下降"=10171] ("starting edge2")
                    w1312 = 10280 items=["上升"=10280, "下降"=10171] ("starting edge1")
                    w1321 = 10171 items=["上升"=10280, "下降"=10171] ("starting edge")
                    w1322 = 10280 items=["上升"=10280, "下降"=10171] ("starting edge")
                    w1323 = 10171 items=["上升"=10280, "下降"=10171] ("starting edge")
                    w1324 = 10280 items=["上升"=10280, "下降"=10171] ("starting edge")
                    n934 = local read "vRES_cCW"() -> (w1320:cluster{dbl[], dbl[]})
                    n935 = Unbundle(w1320) -> (w1317:dbl[], w1315:dbl[])
                    n936 = call "占空比测量.vi"("计数器"=tag "Dev2/ctr6", "starting edge1"=w1324, "starting edge2"=w1323) -> ("占空比2(%)"=w1326:dbl)  [unwired: 4 in, 3 out]
                    n937 = call "占空比测量.vi"("计数器"=tag "Dev2/ctr7", "starting edge1"=w1322, "starting edge2"=w1321) -> ("占空比(%)"=w1325:dbl)  [unwired: 4 in, 3 out]
                    n938 = Reverse 1D Array(array=w1317) -> (reversed array=w1316:dbl[])
                    n939 = Threshold 1D Array(2:315.0 ("分数索引或x"), 3:w1316) -> (0:w1318:dbl)  [unwired: 1 in]
                    n940 = call "Calc_Vres.vi"("S_Data in"=w1325, "P_Data in"=w1326) -> ("Vres"=w1302:dbl)  [unwired: 7 in, 2 out]
                    n941 = Reverse 1D Array(array=w1315) -> (reversed array=w1314:dbl[])
                    n942 = call "占空比测量.vi"("计数器"=tag "Dev2/ctr4", "starting edge1"=w1312, "starting edge2"=w1311) -> ("占空比2(%)"=w1307:dbl)  [unwired: 4 in, 3 out]
                    n943 = call "占空比测量.vi"("计数器"=tag "Dev2/ctr5", "starting edge1"=w1309, "starting edge2"=w1310) -> ("占空比2(%)"=w1306:dbl)  [unwired: 4 in, 3 out]
                    n944 = Interpolate 1D Array(1:w1318, 2:w1314) -> (0:w1303:dbl)
                    n945 = Subtract(x=w1307, y=w1306) -> (x-y=→"T1-T2_315°":dbl)
                    n946 = Max & Min(x=w1302, y=w1303) -> (max(x,y)=w1304:dbl)  [unwired: 1 out]
                    n947 = local write "Vres_315°"(w1304) -> ()
                  }
                  frame #2 {
                    n948 = call "设备状态.vi"("枚举"=enum16{"Read", "Write"}."Write", "工位"=enum16{"工位一", "工位二"}."工位一", "Status_Write"=i16 522) -> ()  [unwired: 8 in, 1 out]
                  }
                }
                n949 = call "浮动通知.vi"("通知内容"="逆向复测！" ("Status")) -> ()  [unwired: 11 in]
              }
              frame 523 {
                n950 = stacked-sequence {
                  frame #0 {
                    n951 = Wait (ms)(milliseconds to wait=u32 500 ("等待时间（毫秒）")) -> ()  [unwired: 1 out]
                  }
                  frame #1 {
                    w1341 = 10171 items=["上升"=10280, "下降"=10171] ("starting edge2")
                    w1340 = 10280 items=["上升"=10280, "下降"=10171] ("starting edge1")
                    w1342 = 10171 items=["上升"=10280, "下降"=10171] ("starting edge2")
                    w1343 = 10280 items=["上升"=10280, "下降"=10171] ("starting edge1")
                    w1352 = 10171 items=["上升"=10280, "下降"=10171] ("starting edge")
                    w1353 = 10280 items=["上升"=10280, "下降"=10171] ("starting edge")
                    w1354 = 10171 items=["上升"=10280, "下降"=10171] ("starting edge")
                    w1355 = 10280 items=["上升"=10280, "下降"=10171] ("starting edge")
                    n952 = local read "vRES_cCW"() -> (w1351:cluster{dbl[], dbl[]})
                    n953 = Unbundle(w1351) -> (w1348:dbl[], w1346:dbl[])
                    n954 = Reverse 1D Array(array=w1348) -> (reversed array=w1347:dbl[])
                    n955 = call "占空比测量.vi"("计数器"=tag "Dev2/ctr6", "starting edge1"=w1355, "starting edge2"=w1354) -> ("占空比2(%)"=w1357:dbl)  [unwired: 4 in, 3 out]
                    n956 = call "占空比测量.vi"("计数器"=tag "Dev2/ctr7", "starting edge1"=w1353, "starting edge2"=w1352) -> ("占空比(%)"=w1356:dbl)  [unwired: 4 in, 3 out]
                    n957 = Threshold 1D Array(2:225.0 ("分数索引或x"), 3:w1347) -> (0:w1349:dbl)  [unwired: 1 in]
                    n958 = Reverse 1D Array(array=w1346) -> (reversed array=w1345:dbl[])
                    n959 = call "Calc_Vres.vi"("S_Data in"=w1356, "P_Data in"=w1357) -> ("Vres"=w1333:dbl)  [unwired: 7 in, 2 out]
                    n960 = Interpolate 1D Array(1:w1349, 2:w1345) -> (0:w1334:dbl)
                    n961 = call "占空比测量.vi"("计数器"=tag "Dev2/ctr4", "starting edge1"=w1343, "starting edge2"=w1342) -> ("占空比2(%)"=w1338:dbl)  [unwired: 4 in, 3 out]
                    n962 = call "占空比测量.vi"("计数器"=tag "Dev2/ctr5", "starting edge1"=w1340, "starting edge2"=w1341) -> ("占空比2(%)"=w1337:dbl)  [unwired: 4 in, 3 out]
                    n963 = Subtract(x=w1338, y=w1337) -> (x-y=→"T1-T2_225°":dbl)
                    n964 = Max & Min(x=w1334, y=w1333) -> (max(x,y)=w1335:dbl)  [unwired: 1 out]
                    n965 = local write "Vres_225°"(w1335) -> ()
                  }
                  frame #2 {
                    n966 = call "设备状态.vi"("枚举"=enum16{"Read", "Write"}."Write", "工位"=enum16{"工位一", "工位二"}."工位一", "Status_Write"=i16 524) -> ()  [unwired: 8 in, 1 out]
                  }
                }
              }
              frame 525 {
                n967 = stacked-sequence {
                  frame #0 {
                    n968 = Wait (ms)(milliseconds to wait=u32 500 ("等待时间（毫秒）")) -> ()  [unwired: 1 out]
                  }
                  frame #1 {
                    w1372 = 10171 items=["上升"=10280, "下降"=10171] ("starting edge2")
                    w1371 = 10280 items=["上升"=10280, "下降"=10171] ("starting edge1")
                    w1373 = 10171 items=["上升"=10280, "下降"=10171] ("starting edge2")
                    w1374 = 10280 items=["上升"=10280, "下降"=10171] ("starting edge1")
                    w1383 = 10171 items=["上升"=10280, "下降"=10171] ("starting edge")
                    w1384 = 10280 items=["上升"=10280, "下降"=10171] ("starting edge")
                    w1385 = 10171 items=["上升"=10280, "下降"=10171] ("starting edge")
                    w1386 = 10280 items=["上升"=10280, "下降"=10171] ("starting edge")
                    n969 = local read "vRES_cCW"() -> (w1382:cluster{dbl[], dbl[]})
                    n970 = Unbundle(w1382) -> (w1377:dbl[], w1379:dbl[])
                    n971 = Reverse 1D Array(array=w1377) -> (reversed array=w1376:dbl[])
                    n972 = call "占空比测量.vi"("计数器"=tag "Dev2/ctr6", "starting edge1"=w1386, "starting edge2"=w1385) -> ("占空比2(%)"=w1388:dbl)  [unwired: 4 in, 3 out]
                    n973 = call "占空比测量.vi"("计数器"=tag "Dev2/ctr7", "starting edge1"=w1384, "starting edge2"=w1383) -> ("占空比(%)"=w1387:dbl)  [unwired: 4 in, 3 out]
                    n974 = Threshold 1D Array(2:135.0 ("分数索引或x"), 3:w1376) -> (0:w1380:dbl)  [unwired: 1 in]
                    n975 = Reverse 1D Array(array=w1379) -> (reversed array=w1378:dbl[])
                    n976 = call "Calc_Vres.vi"("S_Data in"=w1387, "P_Data in"=w1388) -> ("Vres"=w1365:dbl)  [unwired: 7 in, 2 out]
                    n977 = Interpolate 1D Array(1:w1380, 2:w1378) -> (0:w1364:dbl)
                    n978 = call "占空比测量.vi"("计数器"=tag "Dev2/ctr4", "starting edge1"=w1374, "starting edge2"=w1373) -> ("占空比2(%)"=w1369:dbl)  [unwired: 4 in, 3 out]
                    n979 = call "占空比测量.vi"("计数器"=tag "Dev2/ctr5", "starting edge1"=w1371, "starting edge2"=w1372) -> ("占空比2(%)"=w1368:dbl)  [unwired: 4 in, 3 out]
                    n980 = Max & Min(x=w1364, y=w1365) -> (max(x,y)=w1366:dbl)  [unwired: 1 out]
                    n981 = Subtract(x=w1369, y=w1368) -> (x-y=→"T1-T2_135°":dbl)
                    n982 = local write "Vres_135°"(w1366) -> ()
                  }
                  frame #2 {
                    n983 = call "设备状态.vi"("枚举"=enum16{"Read", "Write"}."Write", "工位"=enum16{"工位一", "工位二"}."工位一", "Status_Write"=i16 526) -> ()  [unwired: 8 in, 1 out]
                  }
                }
              }
              frame 527 {
                n984 = stacked-sequence {
                  frame #0 {
                    n985 = Wait (ms)(milliseconds to wait=u32 500 ("等待时间（毫秒）")) -> ()  [unwired: 1 out]
                  }
                  frame #1 {
                    w1401 = 10171 items=["上升"=10280, "下降"=10171] ("starting edge2")
                    w1402 = 10280 items=["上升"=10280, "下降"=10171] ("starting edge1")
                    w1398 = 10171 items=["上升"=10280, "下降"=10171] ("starting edge2")
                    w1399 = 10280 items=["上升"=10280, "下降"=10171] ("starting edge1")
                    w1414 = 10171 items=["上升"=10280, "下降"=10171] ("starting edge")
                    w1415 = 10280 items=["上升"=10280, "下降"=10171] ("starting edge")
                    w1416 = 10171 items=["上升"=10280, "下降"=10171] ("starting edge")
                    w1417 = 10280 items=["上升"=10280, "下降"=10171] ("starting edge")
                    n986 = local read "vRES_cCW"() -> (w1413:cluster{dbl[], dbl[]})
                    n987 = Unbundle(w1413) -> (w1409:dbl[], w1408:dbl[])
                    n988 = call "占空比测量.vi"("计数器"=tag "Dev2/ctr6", "starting edge1"=w1417, "starting edge2"=w1416) -> ("占空比2(%)"=w1419:dbl)  [unwired: 4 in, 3 out]
                    n989 = call "占空比测量.vi"("计数器"=tag "Dev2/ctr7", "starting edge1"=w1415, "starting edge2"=w1414) -> ("占空比(%)"=w1418:dbl)  [unwired: 4 in, 3 out]
                    n990 = Reverse 1D Array(array=w1409) -> (reversed array=w1410:dbl[])
                    n991 = call "Calc_Vres.vi"("S_Data in"=w1418, "P_Data in"=w1419) -> ("Vres"=w1396:dbl)  [unwired: 7 in, 2 out]
                    n992 = Reverse 1D Array(array=w1408) -> (reversed array=w1407:dbl[])
                    n993 = Threshold 1D Array(2:45.0 ("分数索引或x"), 3:w1410) -> (0:w1412:dbl)  [unwired: 1 in]
                    n994 = Interpolate 1D Array(1:w1412, 2:w1407) -> (0:w1395:dbl)
                    n995 = Max & Min(x=w1395, y=w1396) -> (max(x,y)=w1397:dbl)  [unwired: 1 out]
                    n996 = call "占空比测量.vi"("计数器"=tag "Dev2/ctr4", "starting edge1"=w1399, "starting edge2"=w1398) -> ("占空比2(%)"=w1406:dbl)  [unwired: 4 in, 3 out]
                    n997 = call "占空比测量.vi"("计数器"=tag "Dev2/ctr5", "starting edge1"=w1402, "starting edge2"=w1401) -> ("占空比2(%)"=w1405:dbl)  [unwired: 4 in, 3 out]
                    n998 = local write "Vres_45°"(w1397) -> ()
                    n999 = Subtract(x=w1406, y=w1405) -> (x-y=→"T1-T2_45°":dbl)
                  }
                  frame #2 {
                    n1000 = local write "STEP"("复测判定") -> ()
                  }
                }
              }
              frame 530 {
              }
              frame 1024 {
                n1001 = local write "STEP"("退出自动" ("STEP")) -> ()
              }
            }
          }
          frame "不合格" {
            n1002 = Wait (ms)(milliseconds to wait=u32 100 ("等待时间（毫秒）")) -> ()  [unwired: 1 out]
            n1003 = local write "STEP"("等待" ("STEP")) -> ()
            n1004 = call "设备状态.vi"("枚举"=enum16{"Read", "Write"}."Write", "工位"=enum16{"工位一", "工位二"}."工位二", "Status_Write"=i16 400) -> ()  [unwired: 8 in, 1 out]
          }
          frame "报表" {
            n1005 = stacked-sequence {
              frame #0 {
                n1006 = global write "Global.vi" "计时开始"(FALSE ("计时开始")) -> ()
                n1007 = disable-structure shown="禁用" {
                  frame Disabled {
                    n1008 = global read "Global.vi" "产品编号"() -> (w1438:string)
                    n1009 = Concatenate Strings("graph\\" ("名称或相对路径"), w1438, ".hsg" ("字符串")) -> (w1439:string)
                    n1010 = call <vilib>:"Application Directory.vi"() -> ("Application Directory"=w1441:path)
                    n1011 = local read "动优化态前"() -> (w1445:cluster{dbl[], dbl[]}[])
                    n1012 = local read "传感器特性"() -> (w1430:cluster{dbl[], dbl[]}[])
                    n1013 = local read "可信度检测"() -> (w1446:cluster{dbl[], dbl[]}[])
                    n1014 = Build Path "创建路径"(base path=w1441, name or relative path=w1439) -> (appended path=w1434:path)
                    n1015 = Bundle("可信度检测"=w1446, "动优化态前"=w1445, "传感器特性"=w1430) -> (w1444:T10)  [unwired: 1 in]
                    n1016 = Open/Create/Replace File "打开/创建/替换文件"(file path (use dialog)=w1434, operation (0:open)=T5."open or create" ("操作(0:open)")) -> (refnum out=w1432:refnum<file>, error out=w1431:errorcluster)  [unwired: 4 in, 1 out]
                    n1017 = Flatten To JSON "平化至JSON"(anything=w1444, error in (no error)=w1431) -> (JSON string=w1443:string, 11:w1442:errorcluster)  [unwired: 1 in]
                    n1018 = Write to Binary File "写入二进制文件"(file (use dialog)=w1432, data=w1443, error in=w1442) -> (refnum out=w1435:refnum<file>, error out=w1436:errorcluster)  [unwired: 3 in, 1 out]
                    n1019 = Close File(refnum=w1435, error in=w1436) -> ()  [unwired: 2 out]
                  }
                  frame Enabled {
                  }
                }
              }
              frame #1 {
                n1020 = global read "Global.vi" "工位"() -> (w1452:enum16{"左工位", "右工位"})
                n1021 = call "时间秒.vi"() -> ("结果字符串"=w1450:string)  [unwired: 11 in]
                n1022 = global read "Global.vi" "产品编号"() -> (w1448:string)
                n1023 = case shown="\"右工位\"" w1452 {
                  tunnel: [_ "右工位" ("工位名称")] -> w1451
                  frame "左工位", Default {
                  }
                  frame "右工位" {
                  }
                }
                n1024 = call <vilib>:"Space Constant.vi"() -> ("String"=w1449:string)
                n1025 = Concatenate Strings(w1448, w1449, w1450) -> (w1447:string)
                n1026 = global read "Global.vi" "联机模式"() -> (w1456:enum16{"单机", "追溯"})
                n1027 = call "Report.vi"("文件重命名"=TRUE, "文件名称"=w1447, "工位名称"=w1451, "判定结果"="判定结果") -> ("RESULT_VALUE"=w1453:string)  [unwired: 6 in, 1 out]
                n1028 = case shown="\"追溯\"" w1456 {
                  tunnel: w1453 -> [_ w1458]
                  frame "单机", Default {
                  }
                  frame "追溯" {
                    n1029 = global read "Global.vi" "Result"() -> (w1463:refnum<vi>)
                    n1030 = property class="Tbl"(reference=w1463) -> (reference out=w1462:refnum<vi>, "Row Headers[]"=w1460:string[])  [unwired: 1 in, 1 out]
                    n1031 = property class="Tbl"(reference=w1462) -> ("Value"=w1461:string[][])  [unwired: 1 in, 2 out]
                    n1032 = for "For循环" {
                      tunnel: w1461 -> [w1469] mode=indexing
                      tunnel: w1460 -> [w1470] mode=indexing
                      tunnel: [w1467] -> w1459 mode=indexing if=w1468
                      n1033 = Index Array(array=w1469) -> (element=w1471:string)  [unwired: 1 in]
                      n1034 = Build Array (concatenate)(w1470, w1469) -> (w1467:string[])
                      n1035 = case shown="\"\"" w1471 {
                        tunnel: [TRUE FALSE] -> w1468
                        frame Default {
                        }
                        frame "" {
                        }
                      }
                    }
                    n1036 = global read "追溯Global.vi" "DEVICE_ID"() -> (w1465:string)
                    n1037 = global read "追溯Global.vi" "CODE_ID"() -> (w1464:string)
                    n1038 = global read "追溯Global.vi" "USER_ID"() -> (w1466:string)
                    n1039 = call "UPRESULT.vi"("DEVICE_ID"=w1465, "USER_ID"=w1466, "CODE_ID"=w1464, "RESULT_VALUE"=w1458) -> ()  [unwired: 11 in, 1 out]
                    n1040 = call "UPTEST.vi"("Result"=w1459, "CODE_ID"=w1464, "DEVICE_ID"=w1465) -> ()  [unwired: 6 in, 1 out]
                  }
                }
              }
              frame #2 {
                n1041 = local write "STEP"("进入自动" ("STEP")) -> ()
              }
            }
          }
        }
        n1042 = global read "Global.vi" "程序关闭"() -> (w15:bool)
      }
      n1043 = while {
        stop <- w1475 stop-if-true
        n1044 = event shown="[0] 超时" {
          selector: _ -> [_ _ _ _ _ _]
          dyn-events: _ -> [_ _ _ _ _ _]
          timeout: 1000 -> [_ _ _ _ _ _]
          event Timeout {
            n1045 = event-data() -> ()  [unwired: 1 in, 3 out]
            n1046 = call "Obtain Broadcast Events for Registration.vi"() -> ("Already running?"=w1477:bool)  [unwired: 9 in, 2 out]
            n1047 = case shown="真" w1477 {
              frame False {
                n1048 = local write "STEP"("手动" ("STEP")) -> ()
              }
              frame True {
                n1049 = call "错误代码.vi"() -> ("Status_Read"=w1479:u32)  [unwired: 11 in]
                n1050 = feedback #9() -> (w1489:u32)  [unwired: 1 in]
                n1051 = feedback-in #9(w1479) -> ()
                n1052 = case shown="0" w1479 {
                  frame 0 {
                    n1053 = global read "Global.vi" "报警图标"() -> (w1490:refnum<vi>)
                    n1054 = property class="Bool"(reference=w1490, "Visible"=FALSE ("可见")) -> ()  [unwired: 1 in, 2 out]
                  }
                  frame 1, Default {
                    n1055 = global read "Global.vi" "报警图标"() -> (w1493:refnum<vi>)
                    n1056 = property class="Bool"(reference=w1493, "Visible"=TRUE ("可见")) -> ()  [unwired: 1 in, 2 out]
                  }
                }
                n1057 = Greater Or Equal?(x=w1479, y=i16 5000) -> (x >= y?=w1487:bool)
                n1058 = Less?(x=w1479, y=i16 5200) -> (x < y?=w1488:bool)
                n1059 = Equal?(x=w1479, y=w1489) -> (x = y?=w1486:bool)
                n1060 = global read "Global.vi" "报警图标"() -> (w1481:refnum<vi>)
                n1061 = And(x=w1487, y=w1488) -> (x .and. y?=w1480:bool)
                n1062 = property class="Bool"(reference=w1481, "Value"=w1480) -> ()  [unwired: 1 in, 2 out]
                n1063 = Bundle By Name(cluster=errorcluster {"status"=FALSE, "code"=0, "source"=""} ("错误常量"), "status"=w1480, "code"=w1479) -> (w1485:errorcluster)
                n1064 = case shown="假" w1486 {
                  tunnel: w1485 -> [w1494 _]
                  frame False {
                    n1065 = call "报警处理.vi"("错误常量"=w1494) -> ()  [unwired: 9 in, 2 out]
                  }
                  frame True {
                  }
                }
              }
            }
          }
          event Menu Selection (User) {
            n1066 = event-data() -> ("ItemTag"=w1495:string)  [unwired: 1 in, 2 out]
            n1067 = case shown="\"假\", 默认" w1495 {
              frame "假", Default {
              }
              frame "真" {
              }
            }
          }
          event "可信度检测": Scale Range Change {
            n1068 = event-data() -> ("CtlRef"=w1496:refnum<vi>)  [unwired: 1 in]
            n1069 = call "XY_conf备份.vi"("方式"=enum16{"写入", "读取"}."写入", "XY图引用"=w1496) -> ()  [unwired: 3 in, 1 out]
          }
          event Panel Close {
            n1070 = event-data() -> ()  [unwired: 1 in, 4 out]
            n1071 = global write "Global.vi" "程序关闭"(TRUE ("程序关闭")) -> ()
          }
          event "传感器特性": Mouse Enter; "传感器特性": Mouse Leave; "传感器特性": Cursor Move {
            n1072 = event-data() -> ("CtlRef"=w1501:refnum<vi>, "Type"=w1499:T11)  [unwired: 1 in]
            n1073 = call "CursorShow.vi"("nameShow"=TRUE, "Type"=w1499, "Graph"=w1501) -> ()  [unwired: 7 in, 2 out]
          }
          event "传感器特性": Mouse Down {
            n1074 = event-data() -> ("CtlRef"=w1506:refnum<vi>, "Coords"=w1505:T12, "Type"=w1503:T11)  [unwired: 1 in]
            n1075 = invoke class="XYGraph (严格)" method="Map Coords To XY"(reference=w1506, "Coords"=w1505) -> (reference out=w1504:refnum<vi>, "XY"=w1502:cluster{"X":dbl, "Y":dbl})  [unwired: 5 in, 5 out]
            n1076 = call "CursorShow.vi"("游标.游标位置"=w1502, "Type"=w1503, "Graph"=w1504) -> ()  [unwired: 7 in, 2 out]
          }
        }
        n1077 = global read "Global.vi" "程序关闭"() -> (w1475:bool)
      }
    }
  }
